vi "SEC code V4.9.vi"() -> ()   [LabVIEW 2022 SP3]
uses:
  SEC code V3.1/Drivers and Aux files/user.lib/atmcd32d.llb/Shutter_type typedef.ctl
  C:/Users/Benj/Desktop/SEC Software V4.9/EcoChemie.Autolab.Sdk.dll
  EcoChemie.Autolab.Sdk.dll
  SEC code V3.1/Drivers and Aux files/State.ctl
  SEC code V3.1/Drivers and Aux files/SECenumctl.ctl
  SEC code V3.1/Drivers and Aux files/user.lib/atmcd32d.llb/TriggerMode_mode typedef.ctl
  SEC code V3.1/Drivers and Aux files/OSSPEC.ctl
  SEC code V3.1/Drivers and Aux files/OSPEC-enum.ctl
  Labview/IVIUM/IVIUM_remdriver.lvlib
panel:
  out "Current PD 2":dbl
  out "POtential PD 2":dbl
  in  "Tab Control 5":enum32{"AUTOLAB", "IVIUM", "iDUS", "Kymera"}(tab)
  out "current":dbl
  out "Error after autolab connection?":errorcluster
  out "Autolab Connected?":bool
  out "Voltage":dbl format="%#_3e"
  out "PotentialOverload":bool
  out "Bandwidth":i32
  out "CurrentRange":i32
  out "Mode":i32
  out "Measured voltage":dbl
  out "CurrentOverload":bool
  out "Cell on?":bool
  out "current":dbl caption="Current (A)" format="%_4g"
  out "cell on":bool
  out "V (during measurment)":dbl
  out "Potentiostat Status":string
  out "T reached?":bool
  out "Shut down sequence run?":bool
  out "Curent Temp":i32
  in  "Tab Control 4":T1(tab)
  in  "Use autolab?":bool=TRUE
  in  "Embedded Exe File":path=path "C:/Program Files/Metrohm Autolab/Autolab SDK 2.1/Hardware Setup Files/Adk.x"
  in  "Hardware Setup File":path=path "C:/ProgramData/Metrohm Autolab/13.0/HardwareSetup.AUT55157.xml"
  in  "Bandwidth 2":i32(ring)=2 items=["UltraHigh_Speed", "High_Speed", "High_Stability"]
  in  "Start potential (V)":dbl=0.2
  in  "Stop potential (V)":dbl=0.7
  in  "Increment (V)":dbl=0.05
  in  "Default Potential (V)":dbl=0.2
  in  "Wait before \nspectrum (s)":dbl=0.1
  in  "Equilibration \ntime (s)":u32=5
  in  "Reverse Scan\ndirection":bool
  in  "(update and read)":bool
  in  "Tab Control 3":T2(tab)
  in  "Inetegration\n Time (us)":i32=5000
  in  "Continuous \nStrobe Delay (us)":i32
  in  "Number of averages":i32
  in  "Use iDus?":bool
  in  "Return detector \nto room T?":bool
  in  "Init, Cool, read dark,\nOR\nWarm/de-init detector":bool
  in  "Temperature\n(degrees C)":i32=-80
  in  "Number of scans in kinetic cycle":i32=30
  in  "Exposure time (s)":dbl=0.03
  in  "Tab Control 2":T3(tab)
  in  "V 1 time (s)":dbl=10.0
  in  "V off time":dbl=30.0
  in  "Sampling\n delay (s)":dbl
  in  "V 2 time (s)":dbl=20.0
  in  "Run OSPSEC":bool
  in  "Square wave?":bool
  out "OCP I (close to 0)":dbl
  out "OCP":dbl format="%_3f"
  in  "V1 (V)":dbl=0.4
  in  "V2 (V)":dbl=0.8
  in  "Slow sample time (s)":dbl=1500.0
  out "Time during PD":u32
  in  "File Name":string="test-1"
  in  "File Path":path=path "C:/Users/Benj/Documents/test"
  in  "Tab Control":T4(tab)
  out "?":T5(graph)
  out "?":cluster{i32[], dbl[]}(graph)
  out "?":T5(graph)
  out "?":T5(graph)
  out "Current during PD":dbl(graph)=1.602783203125e-06
  out "?":cluster{dbl[], dbl[]}(graph)
  out "Potential  During PD":dbl(graph)=-0.0002471923828124972
  out "Setpoint":dbl
  out "?":cluster{i32[], "array":i32[]}(graph)
  out "I_overload":bool
  out "Aninput1_overload":bool
  out "E_overload":bool
  out "cell-off button pressed":bool
  in  "Default\nCurrent range":T6(ring)=enum."100 uA"
  in  "Default Filter":T7(ring)=enum."10 kHz"
  out "Device serial number":string
  in  "Set Stability":T8(ring)=enum."Standard"
  out "Number of Spectrometers":i32
  out "IDus not in read loop? (kinetic)":bool
  out "Get status return code":dbl
  out "xpixels":i32
  out "ypixels":i32
  out "Calculated exposure time":sgl format="%.2f"
  out "Check timings return code":u32
  out "Set temprature\nreturn code":u32
  out "get aquired data return code":u32
  out "Start Aquisition return code":u32
  out "Init. return code":u32
  out "Cooler Off return code":u32
  out "Time before the start of current aquisition (ms)":u32
  out "Time  after the aquisition (before fetch data), (ms)":u32
  in  "Shutter opens on TTL":T9=enum."TTL High"
  in  "Shutter open and close time":i32
  out "Get aqisition ok? (kinetic mode)":bool
  out "Time taken to apply V2":u32
  out "Values to re-intialise to at end\nof the measument":T10
  out "V2 applied?":bool
  out "ContinuousStrobe Out":u32
  out "Wrapper Out":u32
  out "WL Values":dbl[](array[numeric])
  out "Number of time the OCEAN averaging loop has run -1":i32
  out "Adc":refnum<k24>
  out "Sampler 2":refnum<k24>
  out "Dio":refnum<k24>
  out "Dac":refnum<k24>
  out "instrument":refnum<k24>
  out "Ei":refnum<k24>
  out "AutolabConnection":refnum<k24>
  out "EI status supported for":string[](array[string])
  out "TemperatureOverload":bool
  out "ManualCellSwitch":bool
  out "Oscillation":bool
  out "PD ENDED\nEXIT MEASURMENT":bool=TRUE
  out "Current PD":dbl
  out "POtential PD":dbl
  in  "Exit and disconnect":bool
  # "Program control"
  # "Potential decay control"
  # "Spectrometer control"
  # "System status"
  # "SEC control"
  # "Cell on?"
  # "Use the integration time program in the same folder as this program\nto get the optimum value. For kinetic mode the time resolution is limited \nby integration time"
  # "Unless you know what you are doing keep these at 0.03 and 30"
  # "I overload overload"
  # "off button pressed"
  # "Aninput1 overload"
  # "E overload"
  # "OSPEC loop exit"
  # "Checklist for avoiding errors:\n(1) Light on the IVIUM should be blue with red flashes\nIf the system crahes and the light is red then connect and disconnect in IVUM soft/turn stat off/on\n(2) Maya Pro should read in ocean view/or the get intensity program\nIf maya is not reading connect and disconnect USB.\n(3) If errors persist rrepeat steps 1 + 2 then re-compile code by clicking the\nwhite (run) whilst holding down CRTL + (left) SHIFT\n(4) IF USING THE iDus DO NOT EXIT WITHOUT WARMING CAMERA BACK TO ROOM T,YOU \nWILL DAMAGE IT \n(6) if the IVIUM.dll does not load click broken arrows and \"show error\" until you see the call library function (see blue circles). Double click on this and paste the following into the directory (red circle):   \n%windir%\\Labview\\IVIUM\\IVIUM_remdriver.dll"
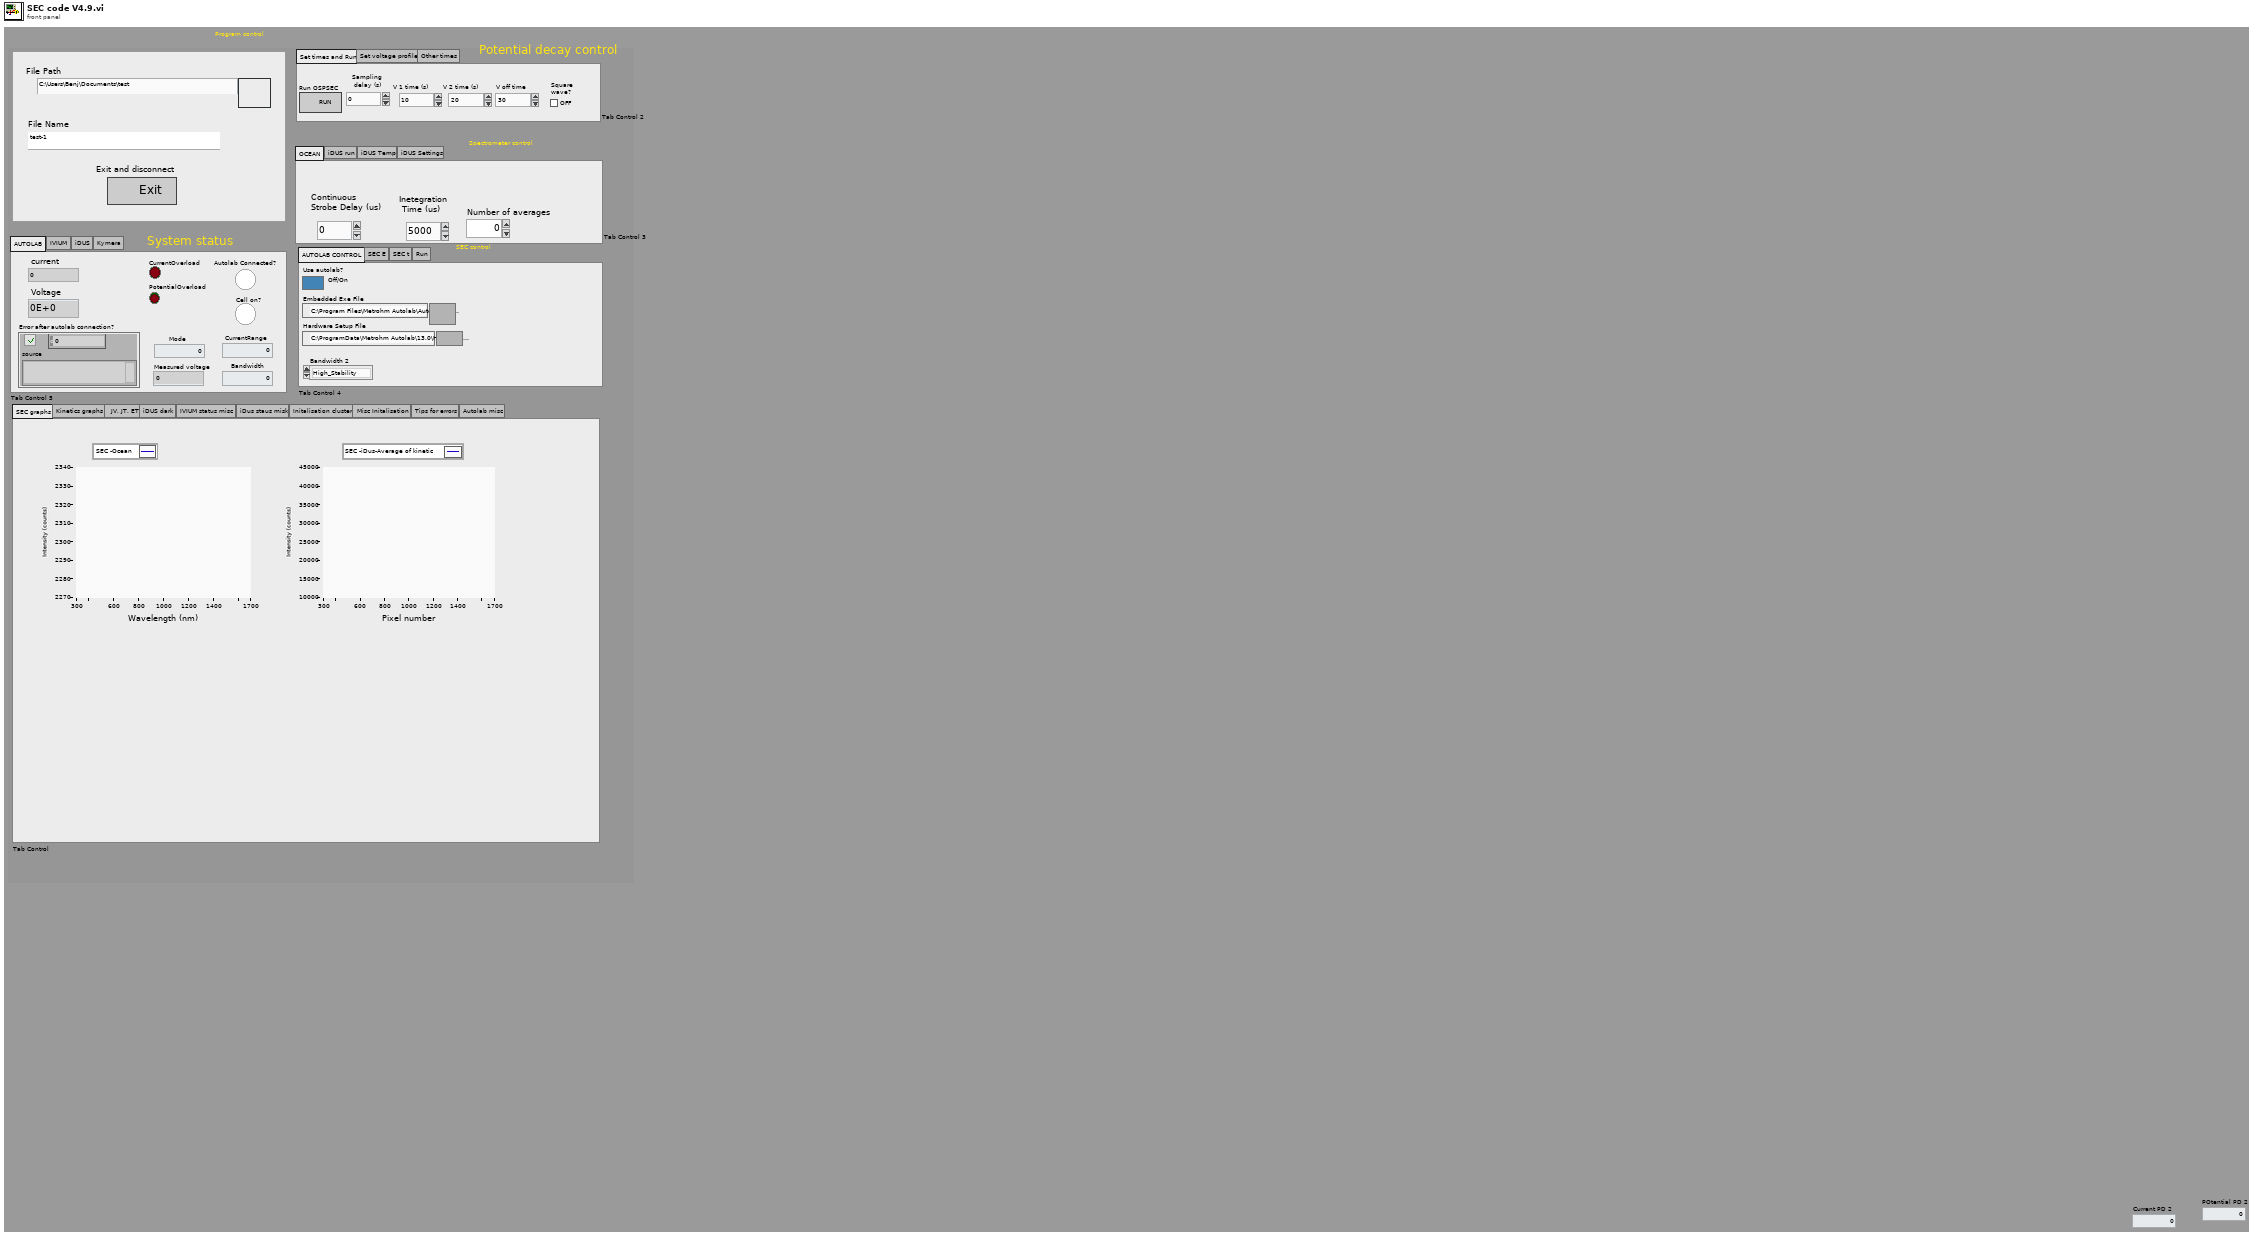
[diagram p1: front panel]
types:
  T1 = enum32{"AUTOLAB CONTROL", "SEC E", "SEC t", "Run"}
  T2 = enum32{"OCEAN", "iDUS run", "iDUS Temp", "iDUS Settings"}
  T3 = enum32{"Set times and Run", "Set voltage profile", "Other times"}
  T4 = enum32{"SEC graphs", "Kinetics graphs", " JV, JT, ET", "iDUS dark", "IVIUM status misc", "iDus staus misk", "Initalisation cluster", "Misc Initalisation ", "Tips for errors", "Autolab misc"}
  T5 = cluster{"WL Values":dbl[], "Spectrum Values":dbl[]}
  T6 = enum16{"10 A", "1 A", "100 mA", "10 mA", "1 mA", "100 uA", "10 uA", "1 uA", "100 nA", "10 nA", "1 nA", "100 pA", "10 pA", "1 pA"}
  T7 = enum16{"1 MHz", "100 kHz", "10 kHz", "1 kHz", "10 Hz"}
  T8 = enum16{"High Speed", "Standard", "High Stability"}
  T9 = typedef "Shutter_type typedef.ctl" = enum16{"TTL Low", "TTL High"}
  T10 = cluster{"Currents":dbl[], "Potentials":dbl[], "Device Status":string, "Device serial no":string, "Current":dbl, "Default \nPotential":dbl, "I overload":bool, "Cell On":bool, "E overload":bool, "Aninput1 overload":bool, "Cell off button pressed":bool, "Start potential":dbl, "Stop potential":dbl, "Increment":dbl, "SEC":dbl[], "Path":path, "File name":string}
  T11 = cluster{"Current array":dbl[], "Potential array":dbl[], "Status":string, "Serial No":string, "Current":dbl, "Default\n potential":dbl, "I overload":bool, "Cell on":bool, "E overload":bool, "Cell of button pressed":bool, "Aninput1 overload":bool, "Stop \npotential":dbl, "Start \npotential":dbl, "Increment":dbl, "Spectrum":dbl[][], "Path":path, "File Name":string, "Sample rate":dbl, "V2 time":dbl, "V off time":dbl, "V 2":dbl, "V 1":dbl, "V1 time":dbl, "Time array":dbl[], "Integration time":i32, "Continous strobe delay":i32, "Time elapsed ":i32, "Start time":i32, "Time for E measurment":i32[], "Time for I measurment ":i32[], "Time for spectrum measurment":i32[], "Return detector to \nroom T":bool, "Number of scans in kinetic cycle":i32, "Exposure time":i32}
  T12 = typedef "State.ctl" = enum16{"Initialize", "Wait for Event", "Run SEC", "Run OSPEC", "Initialse and cool iDus", "Exit"}
  T13 = typedef "SECenumctl.ctl" = enum16{"Read spectrum from Ocean", "Read spectrum from iDus", "Apply potential", "Wait", "Apply potential Autolab"}
  T14 = typedef "TriggerMode_mode typedef.ctl" = enum16{"Internal", "External", "N/A (2)", "N/A (3)", "N/A (4)", "N/A (5)", "External Start", "External Exposure (Bulb)", "N/A (8)", "External FVB EM", "Software", "N/A (11)", "External Charge Shifting"}
  T15 = typedef "OSSPEC.ctl" = enum16{"Read Potential and spectrum", "Read current and spectrum", "Reinitialise Cell", "Apply V1", "End measurment", "Apply V2"}
  T16 = typedef "OSPEC-enum.ctl" = enum16{"Check exit", "Read", "Wait"}
  T17 = enum16{"off", "EStat4EL", "EStat2EL", "EStatDummy1", "EStatDummy2", "EStatDummy3", "EStatDummy4", "IStat4EL", "IStat2EL", "IStatDummy", "BiStat4EL", "BiStat2EL"}
  T18 = typedef "Error Code Enum typedef.ctl" = enum32{"N/A (0)", "DRV_ERROR_CODES", "DRV_SUCCESS", "DRV_VXDNOTINSTALLED", "DRV_ERROR_SCAN", "DRV_ERROR_CHECK_SUM", "DRV_ERROR_FILELOAD", "DRV_UNKNOWN_FUNC", "DRV_ERROR_VXD_INIT", "DRV_ERROR_ADDRESS", "DRV_ERROR_PAGELOCK", "DRV_ERROR_PAGEUNLOCK", "DRV_ERROR_BOARDTEST", "DRV_ERROR_ACK", "DRV_ERROR_UP_FIFO", "DRV_ERROR_PATTERN", "N/A (16)", "DRV_ACQUISITION_ERRORS", "DRV_ACQ_BUFFER", "DRV_ACQ_DOWNFIFO_FULL", "DRV_PROC_UNKONWN_INSTRUCTION", "DRV_ILLEGAL_OP_CODE", "DRV_KINETIC_TIME_NOT_MET", "DRV_ACCUM_TIME_NOT_MET", "DRV_NO_NEW_DATA", "N/A (25)", "DRV_SPOOLERROR", "N/A (27)", "N/A (28)", "N/A (29)", "N/A (30)", "N/A (31)", "N/A (32)", "DRV_TEMPERATURE_CODES", "DRV_TEMPERATURE_OFF", "DRV_TEMPERATURE_NOT_STABILIZED", "DRV_TEMPERATURE_STABILIZED", "DRV_TEMPERATURE_NOT_REACHED", "DRV_TEMPERATURE_OUT_RANGE", "DRV_TEMPERATURE_NOT_SUPPORTED", "DRV_TEMPERATURE_DRIFT", "N/A (41)", "N/A (42)", "N/A (43)", "N/A (44)", "N/A (45)", "N/A (46)", "N/A (47)", "N/A (48)", "DRV_GENERAL_ERRORS", "DRV_INVALID_AUX", "DRV_COF_NOTLOADED", "DRV_FPGAPROG", "DRV_FLEXERROR", "DRV_GPIBERROR", "N/A (55)", "N/A (56)", "N/A (57)", "N/A (58)", "N/A (59)", "N/A (60)", "N/A (61)", "N/A (62)", "N/A (63)", "DRV_DATATYPE", "DRV_DRIVER_ERRORS", "DRV_P1INVALID", "DRV_P2INVALID", "DRV_P3INVALID", "DRV_P4INVALID", "DRV_INIERROR", "DRV_COFERROR", "DRV_ACQUIRING", "DRV_IDLE", "DRV_TEMPCYCLE", "DRV_NOT_INITIALIZED", "DRV_P5INVALID", "DRV_P6INVALID", "DRV_INVALID_MODE", "DRV_INVALID_FILTER", "DRV_I2CERRORS", "DRV_I2CDEVNOTFOUND", "DRV_I2CTIMEOUT", "DRV_P7INVALID", "N/A (84)", "N/A (85)", "N/A (86)", "N/A (87)", "N/A (88)", "N/A (89)", "DRV_IOCERROR", "DRV_VRMVERSIONERROR"}
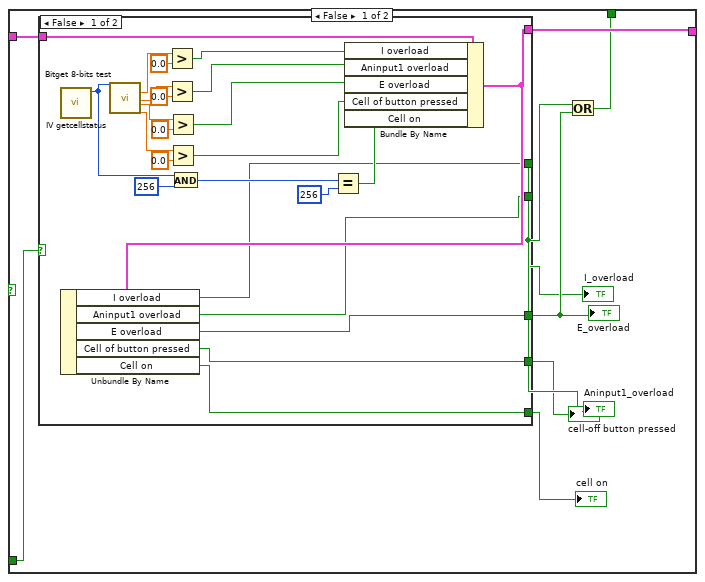
[diagram p2: hidden frame]
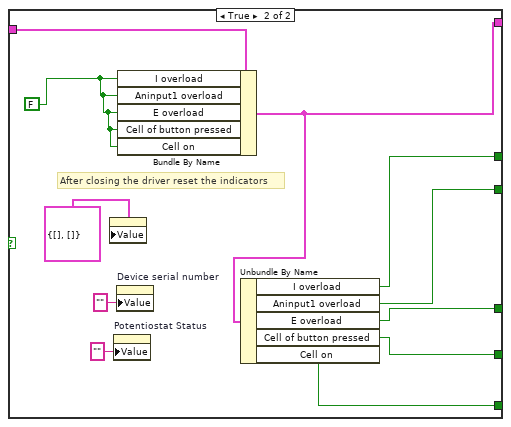
[diagram p3: hidden frame]
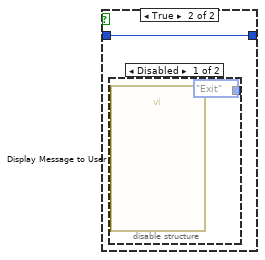
[diagram p4: hidden frame]
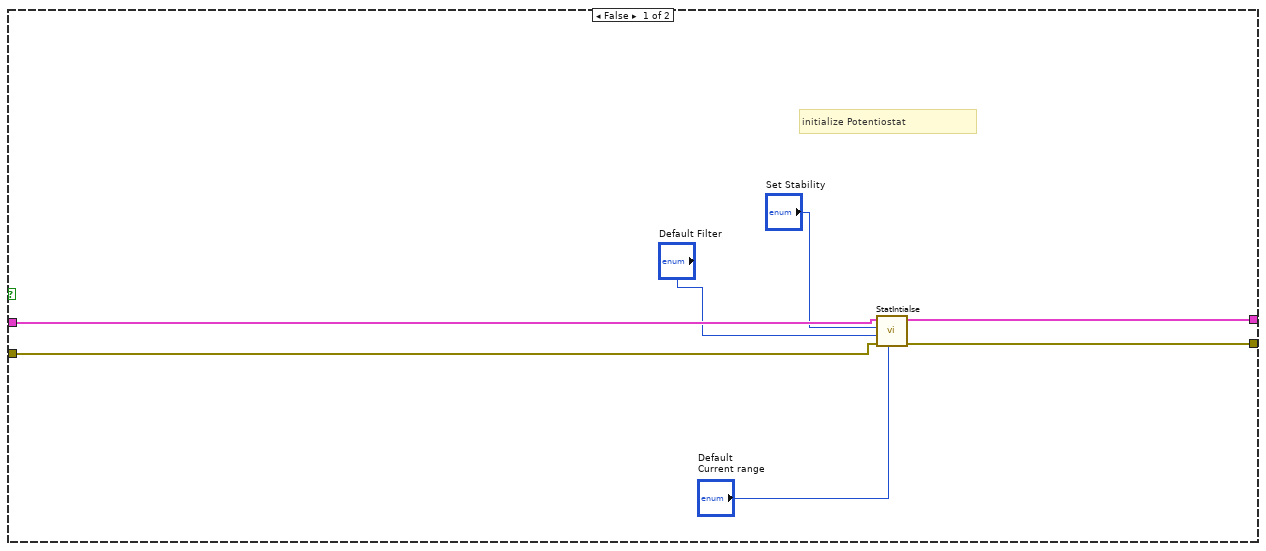
[diagram p7: hidden frame]
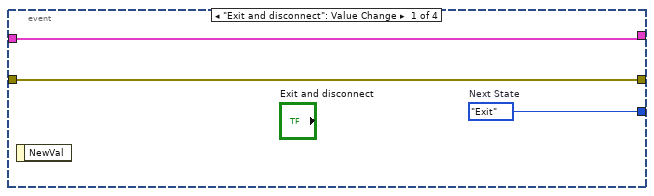
[diagram p9: hidden frame]
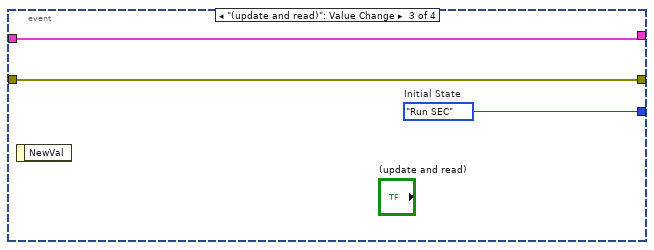
[diagram p10: hidden frame]
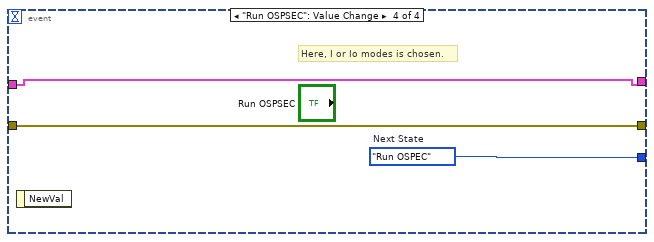
[diagram p11: hidden frame]
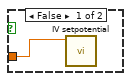
[diagram p12: hidden frame]
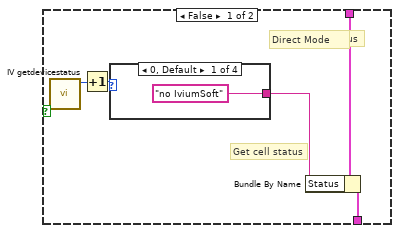
[diagram p13: hidden frame]
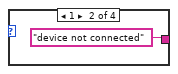
[diagram p14: hidden frame]
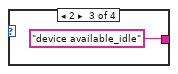
[diagram p15: hidden frame]
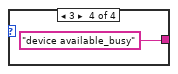
[diagram p16: hidden frame]
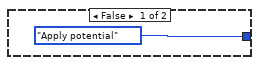
[diagram p17: hidden frame]
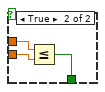
[diagram p20: hidden frame]
diagram:
  w1 = T11 {"Current array"=[], "Potential array"=[], "Status"="", "Serial No"="", "Current"=0.0, "Default\n potential"=0.0, "I overload"=FALSE, "Cell on"=FALSE, "E overload"=FALSE, "Cell of button pressed"=FALSE, "Aninput1 overload"=FALSE, "Stop \npotential"=0.0, "Start \npotential"=0.0, "Increment"=0.0, "Spectrum"=[], "Path"=path "", "File Name"="", "Sample rate"=0.0, "V2 time"=0.0, "V off time"=0.0, "V 2"=0.0, "V 1"=0.0, "V1 time"=0.0, "Time array"=[], "Integration time"=0, "Continous strobe delay"=0, "Time elapsed "=0, "Start time"=0, "Time for E measurment"=[], "Time for I measurment "=[], "Time for spectrum measurment"=[], "Return detector to \nroom T"=FALSE, "Number of scans in kinetic cycle"=0, "Exposure time"=0}  # Init cluster
  w3 = State."Initialize"  # Initial State
  n1 = while {
    shift-right: [w21] -> _
    shift-left: w3 -> [w38]
    shift-right: [w24] -> _
    shift-left: w1 -> [w17]
    shift-right: [w25] -> _
    shift-left: errorcluster {"status"=FALSE, "code"=0, "source"=""} ("error constant") -> [w37]
    stop <- w35 stop-if-true
    # "Main VI State Machine"
    n2 = Bundle By Name(cluster=w17, "Sample rate"="Sampling\n delay (s)", "V1 time"="V 1 time (s)", "V2 time"="V 2 time (s)", "V off time"="V off time", "V 2"="V2 (V)", "V 1"="V1 (V)", "Integration time"="Inetegration\n Time (us)", "Continous strobe delay"="Continuous \nStrobe Delay (us)", "Exposure time"="Exposure time (s)", "Number of scans in kinetic cycle"="Number of scans in kinetic cycle") -> (w11:T11)
    n3 = Bundle By Name(cluster=w11, "Default\n potential"="Default Potential (V)", "Start \npotential"="Start potential (V)", "Stop \npotential"="Stop potential (V)", "Increment"="Increment (V)", "Path"="File Path", "File Name"="File Name") -> (w23:T11)
    n4 = case shown="\"Run SEC\"" w38 {
      tunnel: [w94 w137 w185 w504 w544 w1701] -> w7
      tunnel: [w93 w134 FALSE ("Stop Loop?") w501 FALSE ("Stop Loop?") _] -> w36
      tunnel: w23 -> [w91 w131 w174 w505 w543 w1699]
      tunnel: [w90 w132 w159 w505 w539 w1699] -> w31
      tunnel: w37 -> [w95 w136 w183 w507 w541 w1698]
      tunnel: [w96 w135 w182 w508 w540 w1698] -> w25
      tunnel: [1 ("devconnect") 1 ("devconnect") 1 ("devconnect") w506 1 ("devconnect") 1 ("devconnect")] -> w22
      frame "Initialize" {
        w93 = FALSE  # Stop Loop?
        w94 = State."Wait for Event"  # Next State
        # "Initialize - Initialize variables needed"
        n5 = case shown="True" "Use autolab?" {
          tunnel: [w104 w108] -> w96
          tunnel: w95 -> [w103 _]
          tunnel: w91 -> [w102 w130]
          tunnel: [w98 w130] -> w90
          frame False {
            # "initialize Potentiostat"
            n6 = call "StatIntialse.vi"("Init cluster 2"=w102, "Set Stability"="Set Stability", "Default\n Filter"="Default Filter", "error in (no error)"=w103, "Default\nCurrent range"="Default\nCurrent range") -> ("Init cluster"=w98:T11, "error out"=w104:errorcluster)  [unwired: 4 in]
          }
          frame True {
            w111 = 0 items=["Potentiostatic", "Galvanostatic"] ("Mode")
            w112 = -3 items=["CR07_1A"=0, "CR06_10A"=1, "CR01_100A"=2, "CR00_1000A"=3, "CR05_20A"=20, "CR04_40A"=40, "CR03_50A"=60, "CR02_80A"=80, "CR19_1pA"=-12, "CR18_10pA"=-11, "CR17_100pA"=-10, "CR16_1nA"=-9, "CR15_10nA"=-8, "CR14_100nA"=-7, "CR13_1uA"=-6, "CR12_10uA"=-5, "CR11_100uA"=-4, "CR10_1mA"=-3, "CR09_10mA"=-2, "CR08_100mA"=-1] ("CurrentRange")
            w114 = 1 items=["Off", "On"] ("CellOnOff")
            n7 = call "Connect AutoLab.vi"("Embedded Exe File"="Embedded Exe File", "Hardware Setup File"="Hardware Setup File") -> ("error out"=w119:errorcluster, ".NET Refnum out"=w128:refnum<k24>)  [unwired: 8 in]
            "Error after autolab connection?" <- w119
            n8 = property class="Instrument"(reference=w128, error in=w119) -> (reference out=→"instrument":refnum<k24>, error out=w120:errorcluster, "Adc"=→"Adc":refnum<k24>, "Dac"=→"Dac":refnum<k24>, "Dio"=→"Dio":refnum<k24>, "AutolabConnection"=w116:refnum<k24>, "Ei"=w107:refnum<k24>)
            "AutolabConnection" <- w116
            n9 = property class="AutolabConnection"(reference=w116) -> ("IsConnected"=→"Autolab Connected?":bool)  [unwired: 1 in, 2 out]
            n10 = property class="EI"(reference=w107, error in=w120) -> (reference out=→"Ei":refnum<k24>, error out=w127:errorcluster, "Sampler"=→"Sampler 2":refnum<k24>)
            n11 = property on="Bandwidth 2" class="Ring (strict)"() -> ("Value"=w113:i32)  [unwired: 2 in, 2 out]
            n12 = property on="Default Potential (V)" class="DigNum (strict)"() -> ("Value"=w110:dbl)  [unwired: 2 in, 2 out]
            n13 = Build Array(w120, w127) -> (w121:errorcluster[])
            n14 = Merge Errors(w121) -> (w109:errorcluster)
            n15 = property class="EI"(reference=w107, error in=w109, "Bandwidth"=w113, "CellOnOff"=w114, "CurrentRange"=w112, "Mode"=w111, "Setpoint"=w110) -> (error out=w108:errorcluster, "Current"=w106:dbl, "Potential"=w105:dbl)  [unwired: 1 out]
            n16 = property on="current" class="DigNum (strict)"("Value"=w106) -> ()  [unwired: 2 in, 2 out]
            n17 = property on="Voltage" class="DigNum (strict)"("Value"=w105) -> ()  [unwired: 2 in, 2 out]
          }
        }
        n18 = property on="V2 applied?" class="Bool (strict)"("Value"=FALSE ("V2 applied")) -> ()  [unwired: 2 in, 2 out]
        "Values to re-intialise to at end\nof the measument" <- T10 {"Currents"=[], "Potentials"=[], "Device Status"="", "Device serial no"="", "Current"=0.0, "Default \nPotential"=0.0, "I overload"=FALSE, "Cell On"=FALSE, "E overload"=FALSE, "Aninput1 overload"=FALSE, "Cell off button pressed"=FALSE, "Start potential"=0.0, "Stop potential"=0.0, "Increment"=0.0, "SEC"=[], "Path"=path "", "File name"=""} ("Values to re-intialise to at end\nof the measument")
      }
      frame "Wait for Event" {
        w134 = FALSE  # Stop Loop?
        # "Wait for Event - Use an Event Structure to monitor the user interface for events that run different states of the state machine."
        n19 = event shown="[1] \"Init, Cool, read dark, OR Warm/de-init detector\": Value Change" {
          selector: _ -> [_ _ _ _]
          dyn-events: _ -> [_ _ _ _]
          timeout: _ -> [_ _ _ _]
          tunnel: [w140 State."Initialse and cool iDus" ("Next State") w147 w151] -> w137
          tunnel: w136 -> [w139 w145 w148 w150]
          tunnel: [w139 w145 w148 w150] -> w135
          tunnel: w131 -> [w138 w143 w146 w149]
          tunnel: [w138 w141 w146 w149] -> w132
          event "Exit and disconnect": Value Change {
            w140 = State."Exit"  # Next State
            n20 = event-data() -> ()  [unwired: 1 in, 1 out]
          }
          event "Init, Cool, read dark,\nOR\nWarm/de-init detector": Value Change {
            n21 = event-data() -> ()  [unwired: 1 in, 4 out]
            n22 = Bundle By Name(cluster=w143, "Return detector to \nroom T"="Return detector \nto room T?") -> (w141:T11)
          }
          event "(update and read)": Value Change {
            w147 = State."Run SEC"  # Initial State
            n23 = event-data() -> ()  [unwired: 1 in, 1 out]
          }
          event "Run OSPSEC": Value Change {
            w151 = State."Run OSPEC"  # Next State
            # "Here, I or Io modes is chosen."
            n24 = event-data() -> ()  [unwired: 1 in, 1 out]
          }
        }
      }
      frame "Run SEC" {
        w185 = State."Wait for Event"  # Next State
        n25 = property on="Use autolab?" class="Bool (strict)"() -> ("Value"=w154:bool)  [unwired: 2 in, 2 out]
        n26 = case shown="True" w154 {
          tunnel: w174 -> [w191 w199]
          tunnel: [w190 w199] -> w161
          frame False {
            # "Get cell status"
            # "Get Device Status"
            # "Direct Mode"
            n27 = call "IV getdevicestatus.vi"() -> ("return type"=w193:i32)  [unwired: 10 in, 1 out]
            n28 = Increment(x=w193) -> (x+1=w192:i32)
            n29 = case shown="0, Default" w192 {
              tunnel: ["no IviumSoft" "device not connected" "device available_idle" "device available_busy"] -> w194
              frame 0, Default {
              }
              frame 1 {
              }
              frame 2 {
              }
              frame 3 {
              }
            }
            n30 = Bundle By Name(cluster=w191, "Status"=w194) -> (w190:T11)
          }
          frame True {
          }
        }
        n31 = property on="Use autolab?" class="Bool (strict)"() -> ("Value"=w156:bool)  [unwired: 2 in, 2 out]
        n32 = case shown="True" w156 {
          tunnel: [SECenumctl."Apply potential" SECenumctl."Apply potential Autolab"] -> w181
          frame False {
          }
          frame True {
          }
        }
        n33 = Unbundle By Name(w161) -> ("Increment"=w180:dbl, "Start \npotential"=w184:dbl, "Stop \npotential"=w175:dbl)
        n34 = while {
          shift-right: [w227] -> w158
          shift-left: w161 -> [w228]
          tunnel: w180 -> [w223]
          tunnel: w184 -> [w222]
          shift-right: [w224] -> w182
          shift-left: w183 -> [w225]
          shift-right: [w216] -> _
          shift-left: w181 -> [w220]
          shift-right: [w218] -> w160
          shift-left: dbl[] [0.0] -> [w217]
          shift-right: [w213] -> w164
          shift-left: dbl[] [0.0] -> [w214]
          tunnel: w175 -> [w215]
          shift-right: [w212] -> w173
          shift-left: dbl[][] [] -> [w211]
          tunnel: "Reverse Scan\ndirection" -> [w210]
          tunnel: [w208] -> _
          tunnel: [w208] -> _
          shift-right: [w207] -> _
          shift-left: -3 ("y") -> [w206]
          i -> [w226]
          stop <- w208 stop-if-true
          n35 = case shown="\"Read spectrum from Ocean\"" w220 {
            tunnel: w228 -> [w251 w315 w350 w365 w463]
            tunnel: [w250 w314 w350 w365 w463] -> w227
            tunnel: w226 -> [w264 w324 _ w372 w471]
            tunnel: w225 -> [w261 w306 w346 w374 w472]
            tunnel: [w252 w295 w346 w374 w472] -> w224
            tunnel: w223 -> [w247 w312 _ _ _]
            tunnel: w222 -> [w263 w323 _ _ _]
            tunnel: [w244 w307 w349 w378 w477] -> w221
            tunnel: [w236 w310 w348 w377 w476] -> w219
            tunnel: [w255 w318 w347 w379 w475] -> w218
            tunnel: w217 -> [w256 w319 w347 w379 w475]
            tunnel: [SECenumctl."Wait" SECenumctl."Wait" w351 w360 w459] -> w216
            tunnel: w215 -> [w236 w310 _ _ _]
            tunnel: w214 -> [w254 w317 w342 w380 w473]
            tunnel: [w253 w316 w342 w380 w473] -> w213
            tunnel: [w248 w313 w341 w368 w466] -> w212
            tunnel: w211 -> [w248 w313 w341 w369 w465]
            tunnel: w210 -> [w237 w311 w340 w376 w464]
            tunnel: [w237 w311 w339 w375 w464] -> w209
            tunnel: w206 -> [w235 w305 w337 w362 w460]
            tunnel: [w235 w304 w337 w362 w460] -> w207
            frame "Apply potential", Default {
              # "Here, the while loop iterates three times for every one change of potential. The loop counter is therefore diveded by three, multipled by the increment and then added to the start  potential to give the next potential in the LSV. Potential is applied, then current is read. These go into a build array function . A wait is inclided to alow the sample to equilibriate at the start potential"
              n36 = Divide(x=w264, y=3) -> (x/y=w259:dbl)
              n37 = Multiply(x=w247, y=w259) -> (x*y=w262:dbl)
              n38 = Add(x=w262, y=w263) -> (x+y=w244:dbl)
              "V (during measurment)" <- w244
              n39 = call "IV setpotential.vi"("error in (no error)"=w261, "value"=w244) -> ("error out"=w258:errorcluster)  [unwired: 7 in, 2 out]
              n40 = Equal To 0?(x=w259) -> (x = 0?=w260:bool)
              n41 = case shown="True" w260 {
                tunnel: w258 -> [w274 w276]
                tunnel: [w274 w276] -> w257
                frame False {
                }
                frame True {
                  n42 = Multiply(x=u32 1000, y="Equilibration \ntime (s)") -> (x*y=w275:u32)
                  n43 = Wait (ms)(milliseconds to wait=w275) -> ()  [unwired: 1 out]
                }
              }
              n44 = Equal To 0?(x=w247) -> (x = 0?=w242:bool)
              n45 = Absolute Value(x=w244) -> (abs(x)=w245:dbl)
              n46 = Build Array (concatenate)(w244, w256) -> (w255:dbl[])
              n47 = Greater?(x=w245, y=3.0) -> (0:w243:bool)
              n48 = call "IV getcurrent.vi"("error in (no error)"=w257) -> ("error out"=w240:errorcluster, "value out"=w238:dbl)  [unwired: 8 in, 1 out]
              n49 = Or(x=w242, y=w243) -> (x .or. y?=w241:bool)
              n50 = flat-sequence {
                tunnel: w240 -> [w268]
                tunnel: [w268] -> w239
                tunnel: w238 -> [w267]
                frame #0 {
                  n51 = call "Current ranging routine (SubVI).vi"("Current"=w267) -> ()  [unwired: 11 in]
                  n52 = Wait (ms)(milliseconds to wait=u32 100) -> ()  [unwired: 1 out]
                }
              }
              n53 = case shown="True" w241 {
                frame False {
                }
                frame True {
                  # "abort if E >3 V or\ndelta E =0"
                  n54 = call "IV setcellon.vi"("cellon"=0) -> ("error out"=w272:errorcluster)  [unwired: 8 in, 2 out]
                  n55 = call "IV close.vi"("error in (no error)"=w272) -> ("error out"=w270:errorcluster)  [unwired: 9 in, 1 out]
                  n56 = call "Display Message to User2"("error in (no error)"=w270) -> ("OK"=w273:bool)  [unwired: 9 in, 1 out]
                  n57 = Stop(stop? (T)=w273) -> ()
                }
              }
              n58 = call "IV getcurrent.vi"("error in (no error)"=w239) -> ("error out"=w252:errorcluster, "value out"=w249:dbl)  [unwired: 8 in, 1 out]
              n59 = Bundle By Name(cluster=w251, "Current"=w249) -> (w250:T11)
              n60 = property on="current" class="DigNum (strict)"("Value"=w249) -> ()  [unwired: 2 in, 2 out]
              n61 = Build Array (concatenate)(w249, w254) -> (w253:dbl[])
            }
            frame "Apply potential Autolab" {
              w308 = 1 items=["Off", "On"] ("CellOnOff")
              w303 = 0 items=["Potentiostatic", "Galvanostatic"] ("Mode")
              # "Here, the while loop iterates three times for every one change of potential. The loop counter is therefore diveded by three, multipled by the increment and then added to the start  potential to give the next potential in the LSV. Potential is applied, then current is read. These go into a build array function . A wait is inclided to alow the sample to equilibriate at the start potential"
              n62 = Divide(x=w324, y=3) -> (x/y=w320:dbl)
              n63 = Multiply(x=w312, y=w320) -> (x*y=w322:dbl)
              n64 = Add(x=w322, y=w323) -> (x+y=w307:dbl)
              "Voltage" <- w307
              n65 = property on="Ei" class="Ref (strict)"() -> ("Value"=w282:refnum<k24>)  [unwired: 2 in, 2 out]
              n66 = property class="EI"(reference=w282, error in=w306, "Bandwidth"="Bandwidth 2", "CellOnOff"=w308, "CurrentRange"=w305, "Mode"=w303, "Setpoint"=w307) -> (error out=w287:errorcluster)  [unwired: 1 out]
              n67 = Equal To 0?(x=w320) -> (x = 0?=w321:bool)
              n68 = case shown="False" w321 {
                tunnel: w287 -> [w332 w335]
                tunnel: [w332 w335] -> w299
                frame False {
                }
                frame True {
                  n69 = property on="Equilibration \ntime (s)" class="DigNum (strict)"() -> ("Value"=w333:u32)  [unwired: 2 in, 2 out]
                  n70 = Multiply(x=u32 1000, y=w333) -> (x*y=w334:u32)
                  n71 = Wait (ms)(milliseconds to wait=w334) -> ()  [unwired: 1 out]
                }
              }
              n72 = property on="Sampler 2" class="Ref (strict)"() -> ("Value"=w280:refnum<k24>)  [unwired: 2 in, 2 out]
              n73 = property class="EI"(reference=w282, error in=w287) -> (error out=w286:errorcluster, "EiStatusSupportedFor"=→"EI status supported for":string[])  [unwired: 1 out]
              n74 = invoke class="Sampler" method="Sample"(reference=w280, error in=w287) -> (error out=w285:errorcluster)  [unwired: 1 in, 2 out]
              n75 = Build Array (concatenate)(w307, w319) -> (w318:dbl[])
              n76 = property class="EI"(reference=w282, error in=w299) -> (reference out=w281:refnum<k24>, error out=w298:errorcluster, "Bandwidth"=→"Bandwidth":i32, "CurrentRange"=→"CurrentRange":i32, "Mode"=→"Mode":i32, "Setpoint"=w296:dbl, "Current"=w297:dbl)
              "Measured voltage" <- w296
              n77 = flat-sequence {
                tunnel: w298 -> [w330]
                tunnel: [w330] -> w284
                tunnel: [w329] -> w304
                tunnel: w297 -> [w328]
                tunnel: w296 -> [w327]
                frame #0 {
                  n78 = Wait (ms)(milliseconds to wait=u32 100) -> ()  [unwired: 1 out]
                  n79 = call "Range_selector.vi"("potential"=w327, "current"=w328) -> ("range integer"=w329:i32)  [unwired: 9 in]
                }
              }
              n80 = Merge Errors(w284, w286, w285) -> (w283:errorcluster)
              n81 = call "P_Stat_Status1.vi"("error in (no error)"=w283, ".NET Refnum in"=w281) -> ("error out"=w289:errorcluster, "ManualCellSwitch"=→"ManualCellSwitch":bool, "Oscillation"=→"Oscillation":bool, "TemperatureOverload"=→"TemperatureOverload":bool, "CurrentOverload"=→"CurrentOverload":bool, "Cell"=→"Cell on?":bool)  [unwired: 3 in, 1 out]
              n82 = property class="EI"(reference=w281, error in=w289) -> (error out=w295:errorcluster, "Current"=w279:dbl)  [unwired: 1 out]
              "current" <- w279
              n83 = Bundle By Name(cluster=w315, "Current"=w279) -> (w314:T11)
              n84 = property on="current" class="DigNum (strict)"("Value"=w279) -> ()  [unwired: 2 in, 2 out]
              n85 = Build Array (concatenate)(w279, w317) -> (w316:dbl[])
            }
            frame "Wait" {
              n86 = Multiply(x="Wait before \nspectrum (s)", y=1000.0) -> (x*y=w345:dbl)
              n87 = Wait (ms)(milliseconds to wait=w345) -> ()  [unwired: 1 out]
              n88 = case shown="False" "Use iDus?" {
                tunnel: [SECenumctl."Read spectrum from Ocean" SECenumctl."Read spectrum from iDus"] -> w351
                frame False {
                }
                frame True {
                }
              }
              n89 = case shown="False" w340 {
                selector: w340 -> [w354 w357]
                tunnel: [0.0 1.0] -> w349
                tunnel: [1.0 ("Stop \npotential") 0.0 ("Stop \npotential")] -> w348
                tunnel: [w354 w357] -> w339
                frame False {
                }
                frame True {
                }
              }
            }
            frame "Read spectrum from iDus" {
              n90 = Unbundle By Name(w365) -> ("Exposure time"=w373:i32, "Number of scans in kinetic cycle"=w366:i32)
              n91 = Equal?(x=w372, y=2) -> (x = y?=w370:bool)
              n92 = Multiply(x=1024, y=w366) -> (x*y=w383:i32)
              n93 = stacked-sequence {
                seq-local: [_ _ _ _ _ _ _ _ _ _ w416 _] -> [_ _ _ _ _ _ _ _ _ _ _ w425]
                tunnel: [_ _ _ _ _ _ _ _ _ _ _ w426] -> w381
                tunnel: w366 -> [_ _ _ _ _ w405 _ _ _ _ _ w424]
                tunnel: w383 -> [_ _ _ _ _ _ _ _ _ _ w417 _]
                tunnel: w373 -> [_ _ _ w401 _ _ _ _ _ _ _ _]
                frame #0 {
                  w398 = u16 3  # AcquisitionMode
                  n94 = call "SetAcquisitionMode.vi"("mode"=w398) -> ()  [unwired: 1 in, 2 out]
                }
                frame #1 {
                  w399 = u16 0  # ReadMode
                  n95 = call "SetReadMode.vi"("mode"=w399) -> ()  [unwired: 1 in, 2 out]
                }
                frame #2 {
                  n96 = call "SetTriggerMode.vi"("mode"=TriggerMode_mode_typedef."Internal") -> ()  [unwired: 1 in, 2 out]
                }
                frame #3 {
                  n97 = call "SetExposureTime.vi"("time"=w401) -> ()  [unwired: 1 in, 2 out]
                }
                frame #4 {
                  n98 = call "GetNumberVSSpeeds.vi"() -> ("number"=w404:i32)  [unwired: 3 in, 2 out]
                  n99 = Subtract(x=w404, y=1) -> (x-y=w402:i32)
                  n100 = call "SetVSSpeed.vi"("index"=w402) -> ()  [unwired: 1 in, 2 out]
                }
                frame #5 {
                  n101 = call "SetNumberKinetics.vi"("number"=w405) -> ()  [unwired: 1 in, 2 out]
                }
                frame #6 {
                  w409 = 0  # Auto Shutter
                  n102 = call "SetShutter.vi"("type"=Shutter_type_typedef."TTL High", "mode"=w409, "closingtime"=0, "openingtime"=0) -> ()  [unwired: 10 in, 2 out]
                }
                frame #7 {
                  n103 = call "GetAcquisitionTimings.vi"() -> ("exposure"=w410:sgl)  [unwired: 11 in, 4 out]
                  n104 = property on="Calculated exposure time" class="DigNum (strict)"("Value"=w410) -> ()  [unwired: 2 in, 2 out]
                }
                frame #8 {
                  n105 = call "StartAcquisition.vi"() -> ("DLL error code"=w411:u32)  [unwired: 2 in, 1 out]
                  n106 = property on="Start Aquisition return code" class="DigNum (strict)"("Value"=w411) -> ()  [unwired: 2 in, 2 out]
                }
                frame #9 {
                  n107 = while {
                    stop <- w414 continue-if-true
                    w415 = u16 72  # DRV ACQUIRING
                    n108 = call "GetStatus.vi"() -> ("DLL error code"=→"Get status return code":u32, "status"=w413:T18)  [unwired: 3 in, 1 out]
                    n109 = Equal?(x=w413, y=w415) -> (x = y?=w414:bool)
                  }
                }
                frame #10 {
                  n110 = flat-sequence {
                    tunnel: [w419] -> w418
                    tunnel: w417 -> [w419]
                    tunnel: [w423] -> w416
                    tunnel: w418 -> [w421]
                    frame #0 {
                    }
                    frame #1 {
                      n111 = call "GetAcquiredData.vi"("size"=w421) -> ("DLL error code"=w420:u32, "array"=w423:i32[])  [unwired: 2 in, 1 out]
                      n112 = Equal?(x=20002 ("DRV_SUCCESS"), y=w420) -> ()  [unwired: 1 out]
                      n113 = property on="get aquired data return code" class="DigNum (strict)"("Value"=w420) -> ()  [unwired: 2 in, 2 out]
                    }
                  }
                }
                frame #11 {
                  n114 = for {
                    N: w424 -> [_]
                    shift-right: [w428] -> w426
                    shift-left: i32[][] [] -> [w430]
                    tunnel: w425 -> [w429]
                    i -> [w433]
                    w431 = 1024 ("x")
                    n115 = Multiply(x=w431, y=w433) -> (x*y=w435:i32)
                    n116 = Equal To 0?(x=w433) -> (x = 0?=w434:bool)
                    n117 = Array Subset(array=w429, index=w435, length=w431) -> (w432:i32[])
                    n118 = case shown="False" w434 {
                      tunnel: w432 -> [w437 w440]
                      tunnel: w430 -> [w438 _]
                      tunnel: [w436 w439] -> w428
                      frame False {
                        n119 = Build Array (concatenate)(w438, w437) -> (w436:i32[][])
                      }
                      frame True {
                        n120 = Build Array(w440) -> (w439:i32[][])
                      }
                    }
                  }
                }
              }
              n121 = property on="Use autolab?" class="Bool (strict)"() -> ("Value"=w361:bool)  [unwired: 2 in, 2 out]
              n122 = case shown="True" w361 {
                tunnel: [SECenumctl."Apply potential" SECenumctl."Apply potential Autolab"] -> w360
                frame False {
                }
                frame True {
                }
              }
              n123 = Unbundle By Name(w365) -> ("Number of scans in kinetic cycle"=w367:i32)
              n124 = flat-sequence {
                tunnel: [w446] -> w363
                tunnel: w381 -> [w444]
                tunnel: w367 -> [w443]
                tunnel: [w441] -> w364
                frame #0 {
                  n125 = for {
                    N: 1023 -> [_]
                    tunnel: w444 -> [w451]
                    tunnel: [w452] -> w446 mode=indexing
                    tunnel: w443 -> [w449]
                    tunnel: [w447] -> w441 mode=indexing
                    i -> [w448]
                    n126 = Index Array(array=w451, index (col)=w448) -> (element=w450:i32[])  [unwired: 1 in]
                    n127 = Add Array Elements(numeric array=w450) -> (sum=w453:i32)
                    n128 = Increment(x=w448) -> (x+1=w447:i32)
                    n129 = Divide(x=w453, y=w449) -> (x/y=w452:dbl)
                  }
                  n130 = Bundle(w441, w446) -> (→"?":cluster{i32[], dbl[]})  [unwired: 1 in]
                }
              }
              n131 = case shown="True" w370 {
                tunnel: w369 -> [w388 _]
                tunnel: w363 -> [w387 w390]
                tunnel: [w386 w391] -> w368
                tunnel: w364 -> [_ w389]
                frame False {
                  n132 = Build Array (concatenate)(w388, w387) -> (w386:dbl[][])
                }
                frame True {
                  n133 = Build Array(w389, w390) -> (w391:dbl[][])
                }
              }
              n134 = case shown="False" w376 {
                selector: w376 -> [w392 w395]
                tunnel: [0.0 1.0] -> w378
                tunnel: [1.0 ("Stop \npotential") 0.0 ("Stop \npotential")] -> w377
                tunnel: [w392 w395] -> w375
                frame False {
                }
                frame True {
                }
              }
            }
            frame "Read spectrum from Ocean" {
              # "Building an matric of WL + intensities of multiple expts"
              n135 = Unbundle By Name(w463) -> ("Integration time"=w462:i32, "Continous strobe delay"=w461:i32)
              n136 = Equal?(x=w471, y=2) -> (x = y?=w469:bool)
              n137 = for {
                N: "Number of averages" -> [_]
                tunnel: [w485] -> w474
                tunnel: [w484] -> w468
                tunnel: w462 -> [w483]
                tunnel: w461 -> [w482]
                shift-right: [w479] -> w457
                shift-left: dbl[] [0.0, 0.0, 0.0, 0.0, 0.0, 0.0, 0.0, 0.0, 0.0, 0.0, 0.0, 0.0, 0.0, 0.0, 0.0, 0.0, 0.0, 0.0, 0.0, 0.0, 0.0, 0.0, 0.0, 0.0, 0.0, 0.0, 0.0, 0.0, 0.0, 0.0, 0.0, 0.0, 0.0, 0.0, 0.0, 0.0, 0.0, 0.0, 0.0, 0.0, 0.0, 0.0, 0.0, 0.0, 0.0, 0.0, 0.0, 0.0, 0.0, 0.0, 0.0, 0.0, 0.0, 0.0, 0.0, 0.0, 0.0, 0.0, 0.0, 0.0, 0.0, 0.0, 0.0, 0.0, 0.0, 0.0, 0.0, 0.0, 0.0, 0.0, 0.0, 0.0, 0.0, 0.0, 0.0, 0.0, 0.0, 0.0, 0.0, 0.0, 0.0, 0.0, 0.0, 0.0, 0.0, 0.0, 0.0, 0.0, 0.0, 0.0, 0.0, 0.0, 0.0, 0.0, 0.0, 0.0, 0.0, 0.0, 0.0, 0.0, 0.0, 0.0, 0.0, 0.0, 0.0, 0.0, 0.0, 0.0, 0.0, 0.0, 0.0, 0.0, 0.0, 0.0, 0.0, 0.0, 0.0, 0.0, 0.0, 0.0, 0.0, 0.0, 0.0, 0.0, 0.0, 0.0, 0.0, 0.0, 0.0, 0.0, 0.0, 0.0, 0.0, 0.0, 0.0, 0.0, 0.0, 0.0, 0.0, 0.0, 0.0, 0.0, 0.0, 0.0, 0.0, 0.0, 0.0, 0.0, 0.0, 0.0, 0.0, 0.0, 0.0, 0.0, 0.0, 0.0, 0.0, 0.0, 0.0, 0.0, 0.0, 0.0, 0.0, 0.0, 0.0, 0.0, 0.0, 0.0, 0.0, 0.0, 0.0, 0.0, 0.0, 0.0, 0.0, 0.0, 0.0, 0.0, 0.0, 0.0, 0.0, 0.0, 0.0, 0.0, 0.0, 0.0, 0.0, 0.0, 0.0, 0.0, 0.0, 0.0, 0.0, 0.0, 0.0, 0.0, 0.0, 0.0, 0.0, 0.0, 0.0, 0.0, 0.0, 0.0, 0.0, 0.0, 0.0, 0.0, 0.0, 0.0, 0.0, 0.0, 0.0, 0.0, 0.0, 0.0, 0.0, 0.0, 0.0, 0.0, 0.0, 0.0, 0.0, 0.0, 0.0, 0.0, 0.0, 0.0, 0.0, 0.0, 0.0, 0.0, 0.0, 0.0, 0.0, 0.0, 0.0, 0.0, 0.0, 0.0, 0.0, 0.0, 0.0, 0.0, 0.0, 0.0, 0.0, 0.0, 0.0, 0.0, 0.0, 0.0, 0.0, 0.0, 0.0, 0.0, 0.0, 0.0, 0.0, 0.0, 0.0, 0.0, 0.0, 0.0, 0.0, 0.0, 0.0, 0.0, 0.0, 0.0, 0.0, 0.0, 0.0, 0.0, 0.0, 0.0, 0.0, 0.0, 0.0, 0.0, 0.0, 0.0, 0.0, 0.0, 0.0, 0.0, 0.0, 0.0, 0.0, 0.0, 0.0, 0.0, 0.0, 0.0, 0.0, 0.0, 0.0, 0.0, 0.0, 0.0, 0.0, 0.0, 0.0, 0.0, 0.0, 0.0, 0.0, 0.0, 0.0, 0.0, 0.0, 0.0, 0.0, 0.0, 0.0, 0.0, 0.0, 0.0, 0.0, 0.0, 0.0, 0.0, 0.0, 0.0, 0.0, 0.0, 0.0, 0.0, 0.0, 0.0, 0.0, 0.0, 0.0, 0.0, 0.0, 0.0, 0.0, 0.0, 0.0, 0.0, 0.0, 0.0, 0.0, 0.0, 0.0, 0.0, 0.0, 0.0, 0.0, 0.0, 0.0, 0.0, 0.0, 0.0, 0.0, 0.0, 0.0, 0.0, 0.0, 0.0, 0.0, 0.0, 0.0, 0.0, 0.0, 0.0, 0.0, 0.0, 0.0, 0.0, 0.0, 0.0, 0.0, 0.0, 0.0, 0.0, 0.0, 0.0, 0.0, 0.0, 0.0, 0.0, 0.0, 0.0, 0.0, 0.0, 0.0, 0.0, 0.0, 0.0, 0.0, 0.0, 0.0, 0.0, 0.0, 0.0, 0.0, 0.0, 0.0, 0.0, 0.0, 0.0, 0.0, 0.0, 0.0, 0.0, 0.0, 0.0, 0.0, 0.0, 0.0, 0.0, 0.0, 0.0, 0.0, 0.0, 0.0, 0.0, 0.0, 0.0, 0.0, 0.0, 0.0, 0.0, 0.0, 0.0, 0.0, 0.0, 0.0, 0.0, 0.0, 0.0, 0.0, 0.0, 0.0, 0.0, 0.0, 0.0, 0.0, 0.0, 0.0, 0.0, 0.0, 0.0, 0.0, 0.0, 0.0, 0.0, 0.0, 0.0, 0.0, 0.0, 0.0, 0.0, 0.0, 0.0, 0.0, 0.0, 0.0, 0.0, 0.0, 0.0, 0.0, 0.0, 0.0, 0.0, 0.0, 0.0, 0.0, 0.0, 0.0, 0.0, 0.0, 0.0, 0.0, 0.0, 0.0, 0.0, 0.0, 0.0, 0.0, 0.0, 0.0, 0.0, 0.0, 0.0, 0.0, 0.0, 0.0, 0.0, 0.0, 0.0, 0.0, 0.0, 0.0, 0.0, 0.0, 0.0, 0.0, 0.0, 0.0, 0.0, 0.0, 0.0, 0.0, 0.0, 0.0, 0.0, 0.0, 0.0, 0.0, 0.0, 0.0, 0.0, 0.0, 0.0, 0.0, 0.0, 0.0, 0.0, 0.0, 0.0, 0.0, 0.0, 0.0, 0.0, 0.0, 0.0, 0.0, 0.0, 0.0, 0.0, 0.0, 0.0, 0.0, 0.0, 0.0, 0.0, 0.0, 0.0, 0.0, 0.0, 0.0, 0.0, 0.0, 0.0, 0.0, 0.0, 0.0, 0.0, 0.0, 0.0, 0.0, 0.0, 0.0, 0.0, 0.0, 0.0, 0.0, 0.0, 0.0, 0.0, 0.0, 0.0, 0.0, 0.0, 0.0, 0.0, 0.0, 0.0, 0.0, 0.0, 0.0, 0.0, 0.0, 0.0, 0.0, 0.0, 0.0, 0.0, 0.0, 0.0, 0.0, 0.0, 0.0, 0.0, 0.0, 0.0, 0.0, 0.0, 0.0, 0.0, 0.0, 0.0, 0.0, 0.0, 0.0, 0.0, 0.0, 0.0, 0.0, 0.0, 0.0, 0.0, 0.0, 0.0, 0.0, 0.0, 0.0, 0.0, 0.0, 0.0, 0.0, 0.0, 0.0, 0.0, 0.0, 0.0, 0.0, 0.0, 0.0, 0.0, 0.0, 0.0, 0.0, 0.0, 0.0, 0.0, 0.0, 0.0, 0.0, 0.0, 0.0, 0.0, 0.0, 0.0, 0.0, 0.0, 0.0, 0.0, 0.0, 0.0, 0.0, 0.0, 0.0, 0.0, 0.0, 0.0, 0.0, 0.0, 0.0, 0.0, 0.0, 0.0, 0.0, 0.0, 0.0, 0.0, 0.0, 0.0, 0.0, 0.0, 0.0, 0.0, 0.0, 0.0, 0.0, 0.0, 0.0, 0.0, 0.0, 0.0, 0.0, 0.0, 0.0, 0.0, 0.0, 0.0, 0.0, 0.0, 0.0, 0.0, 0.0, 0.0, 0.0, 0.0, 0.0, 0.0, 0.0, 0.0, 0.0, 0.0, 0.0, 0.0, 0.0, 0.0, 0.0, 0.0, 0.0, 0.0, 0.0, 0.0, 0.0, 0.0, 0.0, 0.0, 0.0, 0.0, 0.0, 0.0, 0.0, 0.0, 0.0, 0.0, 0.0, 0.0, 0.0, 0.0, 0.0, 0.0, 0.0, 0.0, 0.0, 0.0, 0.0, 0.0, 0.0, 0.0, 0.0, 0.0, 0.0, 0.0, 0.0, 0.0, 0.0, 0.0, 0.0, 0.0, 0.0, 0.0, 0.0, 0.0, 0.0, 0.0, 0.0, 0.0, 0.0, 0.0, 0.0, 0.0, 0.0, 0.0, 0.0, 0.0, 0.0, 0.0, 0.0, 0.0, 0.0, 0.0, 0.0, 0.0, 0.0, 0.0, 0.0, 0.0, 0.0, 0.0, 0.0, 0.0, 0.0, 0.0, 0.0, 0.0, 0.0, 0.0, 0.0, 0.0, 0.0, 0.0, 0.0, 0.0, 0.0, 0.0, 0.0, 0.0, 0.0, 0.0, 0.0, 0.0, 0.0, 0.0, 0.0, 0.0, 0.0, 0.0, 0.0, 0.0, 0.0, 0.0, 0.0, 0.0, 0.0, 0.0, 0.0, 0.0, 0.0, 0.0, 0.0, 0.0, 0.0, 0.0, 0.0, 0.0, 0.0, 0.0, 0.0, 0.0, 0.0, 0.0, 0.0, 0.0, 0.0, 0.0, 0.0, 0.0, 0.0, 0.0, 0.0, 0.0, 0.0, 0.0, 0.0, 0.0, 0.0, 0.0, 0.0, 0.0, 0.0, 0.0, 0.0, 0.0, 0.0, 0.0, 0.0, 0.0, 0.0, 0.0, 0.0, 0.0, 0.0, 0.0, 0.0, 0.0, 0.0, 0.0, 0.0, 0.0, 0.0, 0.0, 0.0, 0.0, 0.0, 0.0, 0.0, 0.0, 0.0, 0.0, 0.0, 0.0, 0.0, 0.0, 0.0, 0.0, 0.0, 0.0, 0.0, 0.0, 0.0, 0.0, 0.0, 0.0, 0.0, 0.0, 0.0, 0.0, 0.0, 0.0, 0.0, 0.0, 0.0, 0.0, 0.0, 0.0, 0.0, 0.0, 0.0, 0.0, 0.0, 0.0, 0.0, 0.0, 0.0, 0.0, 0.0, 0.0, 0.0, 0.0, 0.0, 0.0, 0.0, 0.0, 0.0, 0.0, 0.0, 0.0, 0.0, 0.0, 0.0, 0.0, 0.0, 0.0, 0.0, 0.0, 0.0, 0.0, 0.0, 0.0, 0.0, 0.0, 0.0, 0.0, 0.0, 0.0, 0.0, 0.0, 0.0, 0.0, 0.0, 0.0, 0.0, 0.0, 0.0, 0.0, 0.0, 0.0, 0.0, 0.0, 0.0, 0.0, 0.0, 0.0, 0.0, 0.0, 0.0, 0.0, 0.0, 0.0, 0.0, 0.0, 0.0, 0.0, 0.0, 0.0, 0.0, 0.0, 0.0, 0.0, 0.0, 0.0, 0.0, 0.0, 0.0, 0.0, 0.0, 0.0, 0.0, 0.0, 0.0, 0.0, 0.0, 0.0, 0.0, 0.0, 0.0, 0.0, 0.0, 0.0, 0.0, 0.0, 0.0, 0.0, 0.0, 0.0, 0.0, 0.0, 0.0, 0.0, 0.0, 0.0, 0.0, 0.0, 0.0, 0.0, 0.0, 0.0, 0.0, 0.0, 0.0, 0.0, 0.0, 0.0, 0.0, 0.0, 0.0, 0.0, 0.0, 0.0, 0.0, 0.0, 0.0, 0.0, 0.0, 0.0, 0.0] -> [w480]
                i -> [w478]
                n138 = call "ReadSpectrum(SubVI).vi"("Continuous \nStrobe Delay"=w482, "Enter the \nInetegration Time"=w483) -> ("Spectrum Values"=w481:dbl[], "WL Values"=w484:dbl[], "Number of Spectrometers"=w485:i32)  [unwired: 7 in]
                n139 = Add(x=w481, y=w480) -> (x+y=w479:dbl[])
                "Number of time the OCEAN averaging loop has run -1" <- w478
              }
              "Number of Spectrometers" <- w474
              n140 = Divide(x=w457, y="Number of averages") -> (x/y=w456:dbl[])
              n141 = case shown="False" w469 {
                tunnel: w468 -> [_ w497]
                tunnel: w456 -> [w493 w496]
                tunnel: [w492 w495] -> w466
                tunnel: w465 -> [w494 _]
                frame False {
                  # "Matrix + int on i >3"
                  n142 = Build Array (concatenate)(w494, w493) -> (w492:dbl[][])
                }
                frame True {
                  # "WL + Int on =3"
                  n143 = Build Array(w497, w496) -> (w495:dbl[][])
                }
              }
              n144 = Bundle("WL Values"=w468, w456) -> (→"?":cluster{"WL Values":dbl[], dbl[]})  [unwired: 1 in]
              n145 = property on="Use autolab?" class="Bool (strict)"() -> ("Value"=w458:bool)  [unwired: 2 in, 2 out]
              n146 = case shown="True" w458 {
                tunnel: [SECenumctl."Apply potential" SECenumctl."Apply potential Autolab"] -> w459
                frame False {
                }
                frame True {
                }
              }
              n147 = case shown="False" w464 {
                tunnel: [0.0 1.0] -> w477
                tunnel: [1.0 ("Stop \npotential") 0.0 ("Stop \npotential")] -> w476
                frame False {
                }
                frame True {
                }
              }
            }
          }
          n148 = case shown="False" w209 {
            tunnel: w221 -> [w231 w233]
            tunnel: w219 -> [w230 w232]
            tunnel: [w229 w234] -> w208
            frame False {
              n149 = Greater Or Equal?(x=w231, y=w230) -> (x >= y?=w229:bool)
            }
            frame True {
              n150 = Less Or Equal?(x=w233, y=w232) -> (x <= y?=w234:bool)
            }
          }
        }
        n151 = Unbundle By Name(w158) -> ("Default\n potential"=w179:dbl)
        n152 = property on="Use autolab?" class="Bool (strict)"() -> ("Value"=w153:bool)  [unwired: 2 in, 2 out]
        n153 = Insert Into Array(array=w160, index=0, new element=0.0 ("new element/subarray")) -> (w169:dbl[])
        n154 = Transpose Matrix(1:w173) -> (0:w172:dbl[][])
        n155 = Bundle(w160, w164) -> (→"?":cluster{dbl[], dbl[]})  [unwired: 1 in]
        n156 = Reverse 1D Array(array=w169) -> (reversed array=w168:dbl[])
        n157 = property on="V (during measurment)" class="DigNum (strict)"("Value"=w179) -> ()  [unwired: 2 in, 2 out]
        n158 = case shown="True" w153 {
          tunnel: w179 -> [w187 w189]
          frame False {
            n159 = call "IV setpotential.vi"("value"=w187) -> ()  [unwired: 8 in, 3 out]
          }
          frame True {
            n160 = property on="Ei" class="Ref (strict)"() -> ("Value"=w188:refnum<k24>)  [unwired: 2 in, 2 out]
            n161 = property class="EI"(reference=w188, "Setpoint"=w189) -> ()  [unwired: 1 in, 2 out]
          }
        }
        n162 = Replace Array Subset(array=w172, new element=w168, index (row)=0 ("index")) -> (w157:dbl[][])  [unwired: 1 in]
        n163 = Bundle By Name(cluster=w158, "Spectrum"=w172, "Current array"=w164, "Potential array"=w160) -> (w159:T11)
        n164 = Build Array(w160, w164) -> (w171:dbl[][])
        n165 = disable-structure shown="Enabled" {
          disable-tunnel: w157 -> [w205 _]
          disable-tunnel: w158 -> [w204 _]
          frame Enabled {
            n166 = call "WriteSEC.vi"("Init cluster"=w204, "Array"=w205) -> ()  [unwired: 10 in]
          }
          frame Disabled {
          }
        }
        n167 = Transpose Matrix(1:w171) -> (0:w170:dbl[][])
        n168 = disable-structure shown="Enabled" {
          disable-tunnel: w170 -> [w203 _]
          disable-tunnel: w159 -> [w202 _]
          frame Enabled {
            n169 = call "Write_JV.vi"("Init cluster"=w202, "Array"=w203) -> ()  [unwired: 10 in]
          }
          frame Disabled {
          }
        }
      }
      frame "Exit" {
        w501 = TRUE  # Stop Loop?
        w504 = State."Exit"  # (Value Not Used)
        # "Switch cell on/off"
        # "Diconnect device and close Ivium remdriver"
        # "Disconnect Ivium device (when connected)\nbefore terminating this VI"
        # "Exit - Exit the application."
        n170 = property on="Shut down sequence run?" class="Bool (strict)"("Value"=FALSE ("Shut down sequence run?")) -> ()  [unwired: 2 in, 2 out]
        n171 = property on="PotentialOverload" class="Bool (strict)"("Value"=FALSE ("PotentialOverload")) -> ()  [unwired: 2 in, 2 out]
        n172 = property on="T reached?" class="Bool (strict)"("Value"=FALSE ("T reached?")) -> ()  [unwired: 2 in, 2 out]
        n173 = property on="Use autolab?" class="Bool (strict)"() -> ("Value"=w502:bool)  [unwired: 2 in, 2 out]
        n174 = case shown="True" w502 {
          tunnel: [w516 w534] -> w508
          tunnel: w507 -> [w513 w529]
          tunnel: [w511 0 ("devconnect")] -> w506
          frame False {
            w509 = FALSE ("Shut down sequence run?")
            # "This re-initialises a display for the iDus camera"
            # "On"
            # "Close Ivium Driver"
            n175 = To Long Integer(number=0) -> (32bit integer=w515:i32)
            n176 = call "IV setcellon.vi"("error in (no error)"=w513, "cellon"=w515) -> ("error out"=w512:errorcluster)  [unwired: 7 in, 2 out]
            n177 = call "IV getdevicestatus.vi"("error in (no error)"=w512) -> ("error out"=w517:errorcluster, "return type"=w518:i32)  [unwired: 9 in]
            n178 = Greater Than 0?(x=w518) -> (x > 0?=w510:bool)
            n179 = case shown="False" w510 {
              tunnel: [w521 w523] -> w519
              tunnel: w517 -> [w521 _]
              tunnel: [0 ("devconnect") w522] -> w511
              frame False {
              }
              frame True {
                w522 = 0 ("devconnect")
                n180 = call "IV connect.vi"("devconnect"=w522) -> ("error out"=w523:errorcluster)  [unwired: 8 in, 2 out]
              }
            }
            n181 = property on="Shut down sequence run?" class="Bool (strict)"("Value"=w509) -> ()  [unwired: 2 in, 2 out]
            n182 = property on="Return detector \nto room T?" class="Bool (strict)"("Value"=w509) -> ()  [unwired: 2 in, 2 out]
            n183 = call "IV close.vi"("error in (no error)"=w519) -> ("error out"=w516:errorcluster)  [unwired: 9 in, 1 out]
          }
          frame True {
            w528 = 0 items=["Off", "On"] ("CellOnOff")
            n184 = property on="Ei" class="Ref (strict)"() -> ("Value"=w527:refnum<k24>)  [unwired: 2 in, 2 out]
            n185 = property class="EI"(reference=w527, error in=w529, "CellOnOff"=w528) -> (error out=w526:errorcluster)  [unwired: 1 out]
            n186 = property on="ManualCellSwitch" class="Bool (strict)"("Value"=FALSE ("ManualCellSwitch")) -> ()  [unwired: 2 in, 2 out]
            n187 = property on="Cell on?" class="Bool (strict)"("Value"=FALSE ("Cell")) -> ()  [unwired: 2 in, 2 out]
            n188 = property on="instrument" class="Ref (strict)"(error in=w526) -> (error out=w532:errorcluster, "Value"=w533:refnum<k24>)  [unwired: 1 in, 1 out]
            n189 = property on="Autolab Connected?" class="Bool (strict)"("Value"=FALSE ("IsConnected")) -> ()  [unwired: 2 in, 2 out]
            n190 = invoke class="Instrument" method="Disconnect"(reference=w533, error in=w532) -> (error out=w534:errorcluster)  [unwired: 1 in, 2 out]
          }
        }
        n191 = property on="V2 applied?" class="Bool (strict)"("Value"=FALSE ("V2 applied")) -> ()  [unwired: 2 in, 2 out]
      }
      frame "Run OSPEC" {
        n192 = property on="Use autolab?" class="Bool (strict)"() -> ("Value"=w536:bool)  [unwired: 2 in, 2 out]
        n193 = case shown="True" w536 {
          tunnel: w543 -> [w549 w557]
          tunnel: [w548 w557] -> w542
          frame False {
            # "Get cell status"
            # "Get Device Status"
            # "Direct Mode"
            n194 = call "IV getdevicestatus.vi"() -> ("return type"=w552:i32)  [unwired: 10 in, 1 out]
            n195 = Increment(x=w552) -> (x+1=w551:i32)
            n196 = case shown="0, Default" w551 {
              tunnel: ["no IviumSoft" "device not connected" "device available_idle" "device available_busy"] -> w550
              frame 0, Default {
              }
              frame 1 {
              }
              frame 2 {
              }
              frame 3 {
              }
            }
            n197 = Bundle By Name(cluster=w549, "Status"=w550) -> (w548:T11)
          }
          frame True {
          }
        }
        n198 = while {
          shift-right: [w558] -> w540
          shift-left: w541 -> [w563]
          shift-right: [w559] -> w539
          shift-left: w542 -> [w565]
          shift-right: [w562] -> _
          shift-left: OSSPEC."Apply V1" -> [w564]
          i -> [w561]
          stop <- w560 stop-if-true
          n199 = case shown="\"Read current and spectrum\"" w564 {
            tunnel: w565 -> [w569 w956 w1471 w1495 w1557 w1620]
            tunnel: w563 -> [w568 w972 w1475 w1494 w1567 w1648]
            tunnel: [OSSPEC."End measurment" w988 OSSPEC."Read Potential and spectrum" OSSPEC."Read current and spectrum" OSSPEC."Read current and spectrum" OSSPEC."End measurment"] -> w562
            tunnel: [w574 w971 w1474 w1490 w1558 w1646] -> w558
            tunnel: [w575 w979 w1471 w1491 w1557 w1620] -> w559
            tunnel: w561 -> [_ _ _ _ _ _]
            tunnel: [FALSE FALSE FALSE FALSE FALSE w1647] -> w560
            frame "Read Potential and spectrum", Default {
              n200 = property on="Use autolab?" class="Bool (strict)"() -> ("Value"=w566:bool)  [unwired: 2 in, 2 out]
              n201 = disable-structure shown="Enabled" {
                disable-tunnel: w568 -> [w590 _]
                disable-tunnel: [w589 _] -> w567
                disable-tunnel: w566 -> [w588 _]
                frame Enabled {
                  n202 = case shown="True" w588 {
                    tunnel: w590 -> [w592 w604]
                    tunnel: [w591 w602] -> w589
                    frame False {
                      n203 = flat-sequence {
                        tunnel: w592 -> [w595]
                        tunnel: [w595] -> w593
                        tunnel: [w596] -> w591
                        tunnel: w593 -> [w597]
                        frame #0 {
                          n204 = Wait (ms)(milliseconds to wait=u32 50) -> ()  [unwired: 1 out]
                        }
                        frame #1 {
                          n205 = To Long Integer(number=T17."IStat4EL" ("Configuration")) -> (32bit integer=w599:i32)
                          n206 = call "IV setconnectionmode.vi"("error in (no error)"=w597, "value"=w599) -> ("error out"=w596:errorcluster)  [unwired: 7 in, 2 out]
                        }
                      }
                    }
                    frame True {
                      w600 = 0 items=["Off", "On"] ("CellOnOff")
                      w605 = -6 items=["CR07_1A"=0, "CR06_10A"=1, "CR01_100A"=2, "CR00_1000A"=3, "CR05_20A"=20, "CR04_40A"=40, "CR03_50A"=60, "CR02_80A"=80, "CR19_1pA"=-12, "CR18_10pA"=-11, "CR17_100pA"=-10, "CR16_1nA"=-9, "CR15_10nA"=-8, "CR14_100nA"=-7, "CR13_1uA"=-6, "CR12_10uA"=-5, "CR11_100uA"=-4, "CR10_1mA"=-3, "CR09_10mA"=-2, "CR08_100mA"=-1] ("CurrentRange")
                      w606 = 0 items=["Potentiostatic", "Galvanostatic"] ("Mode")
                      n207 = property on="Ei" class="Ref (strict)"() -> ("Value"=w601:refnum<k24>)  [unwired: 2 in, 2 out]
                      n208 = property class="EI"(reference=w601, error in=w604, "CurrentRange"=w605) -> (error out=w603:errorcluster)  [unwired: 1 out]
                      n209 = property class="EI"(reference=w601, error in=w603, "Mode"=w606, "CellOnOff"=w600) -> (error out=w602:errorcluster)  [unwired: 1 out]
                    }
                  }
                }
                frame Disabled {
                }
              }
              n210 = Unbundle By Name(w569) -> ("Spectrum"=w577:dbl[][])
              n211 = Unbundle By Name(w569) -> ("Time for spectrum measurment"=w576:i32[], "Start time"=w579:i32)
              n212 = Unbundle By Name(w569) -> ("Potential array"=w572:dbl[])
              n213 = property on="Use iDus?" class="Bool (strict)"() -> ("Value"=w570:bool)  [unwired: 2 in, 2 out]
              n214 = Unbundle By Name(w569) -> ("Time for E measurment"=w571:i32[], "Start time"=w578:i32)
              n215 = while {
                shift-right: [w838] -> _
                shift-left: w569 -> [w839]
                shift-right: [w830] -> _
                shift-left: OSPEC-enum."Wait" -> [w840]
                shift-right: [w837] -> w582
                shift-left: w571 -> [w836]
                shift-right: [w831] -> w581
                shift-left: w572 -> [w834]
                shift-right: [w833] -> _
                shift-left: w578 -> [w832]
                shift-right: [w828] -> w574
                shift-left: w567 -> [w829]
                i -> [w835]
                stop <- w825 stop-if-true
                n216 = case shown="\"Read\", Default" w840 {
                  tunnel: w839 -> [w848 w859 w950]
                  tunnel: [w848 w859 w950] -> w838
                  tunnel: [w847 FALSE FALSE] -> w827
                  tunnel: [w852 w863 w948] -> w837
                  tunnel: w836 -> [w852 w864 w948]
                  tunnel: w835 -> [_ w868 _]
                  tunnel: [w850 w867 w945] -> w831
                  tunnel: w834 -> [w850 w866 w945]
                  tunnel: [w843 w860 w947] -> w833
                  tunnel: w832 -> [w843 _ w947]
                  tunnel: [OSPEC-enum."Wait" OSPEC-enum."Check exit" OSPEC-enum."Read"] -> w830
                  tunnel: w829 -> [w849 w856 w944]
                  tunnel: [w849 w855 w944] -> w828
                  frame "Check exit" {
                    n217 = Unbundle By Name(w848) -> ("V off time"=w845:dbl)
                    n218 = Multiply(x=w845, y=1000.0) -> (x*y=w846:dbl)
                    n219 = Greater Or Equal?(x=w843, y=w846) -> (x >= y?=w847:bool)
                  }
                  frame "Read", Default {
                    # "Building a 1d matrix of potentials and times"
                    n220 = property on="Use autolab?" class="Bool (strict)"() -> ("Value"=w853:bool)  [unwired: 2 in, 2 out]
                    n221 = case shown="True" w853 {
                      tunnel: [w871 w874] -> w857
                      tunnel: w856 -> [w870 w872]
                      tunnel: [w869 w873] -> w855
                      frame False {
                        n222 = call "IV getpotential.vi"("error in (no error)"=w870) -> ("error out"=w869:errorcluster, "value out"=w871:dbl)  [unwired: 8 in, 1 out]
                      }
                      frame True {
                        n223 = disable-structure shown="Enabled" {
                          disable-tunnel: [w879 _ w925] -> w874
                          disable-tunnel: [w878 _ w927] -> w873
                          disable-tunnel: w872 -> [w876 _ w935]
                          frame Disabled {
                            n224 = property on="Ei" class="Ref (strict)"() -> ("Value"=w877:refnum<k24>)  [unwired: 2 in, 2 out]
                            n225 = disable-structure shown="Enabled" {
                              disable-tunnel: w877 -> [w887 _]
                              disable-tunnel: w876 -> [w883 w888]
                              disable-tunnel: [w882 w888] -> w875
                              frame Disabled {
                                w884 = -4 items=["CR07_1A"=0, "CR06_10A"=1, "CR01_100A"=2, "CR00_1000A"=3, "CR05_20A"=20, "CR04_40A"=40, "CR03_50A"=60, "CR02_80A"=80, "CR19_1pA"=-12, "CR18_10pA"=-11, "CR17_100pA"=-10, "CR16_1nA"=-9, "CR15_10nA"=-8, "CR14_100nA"=-7, "CR13_1uA"=-6, "CR12_10uA"=-5, "CR11_100uA"=-4, "CR10_1mA"=-3, "CR09_10mA"=-2, "CR08_100mA"=-1] ("CurrentRange")
                                w886 = 1 items=["Potentiostatic", "Galvanostatic"] ("Mode")
                                n226 = property class="EI"(reference=w887, error in=w883, "Mode"=w886, "Setpoint"=0.0, "CurrentRange"=w884) -> (error out=w882:errorcluster)  [unwired: 1 out]
                              }
                              frame Enabled {
                              }
                            }
                            n227 = property class="EI"(reference=w877, error in=w875) -> (error out=w878:errorcluster, "Current"=w880:dbl, "Potential"=w879:dbl)  [unwired: 1 out]
                            n228 = disable-structure shown="Enabled" {
                              disable-tunnel: w880 -> [w881 _]
                              frame Disabled {
                                "OCP I (close to 0)" <- w881
                              }
                              frame Enabled {
                              }
                            }
                          }
                          frame Disabled {
                            n229 = property on="Property Node" class="Ref (strict)"() -> ("Value"=w890:refnum<k24>)  [unwired: 2 in, 2 out]
                            n230 = disable-structure shown="Disabled" {
                              disable-tunnel: _ -> [w916 _]
                              disable-tunnel: [w915 _] -> _
                              disable-tunnel: _ -> [w912 _]
                              disable-tunnel: w890 -> [w911 _]
                              frame Disabled {
                                w909 = 2 items=["UltraHigh_Speed", "High_Speed", "High_Stability"] ("Bandwidth")
                                w914 = 1 items=["Off", "On"] ("CellOnOff")
                                w910 = 0 items=["Potentiostatic", "Galvanostatic"] ("Mode")
                                n231 = property on="Property Node" class="Ring (strict)"() -> ("Value"=w913:i32)  [unwired: 2 in, 2 out]
                                n232 = property class="EI"(reference=w911, error in=w912, "Bandwidth"=w909, "CellOnOff"=w914, "CurrentRange"=w913, "Mode"=w910, "Setpoint"=w916) -> (error out=w915:errorcluster)  [unwired: 1 out]
                                n233 = property on="Property Node" class="Ref (strict)"(error in=w915) -> (error out=w908:errorcluster, "Value"=w905:refnum<k24>)  [unwired: 1 in, 1 out]
                                n234 = property class="EI"(reference=w911, error in=w915) -> (error out=w906:errorcluster, "EiStatusSupportedFor"=w907:string[])  [unwired: 1 out]
                                n235 = invoke class="Sampler" method="Sample"(reference=w905, error in=w908) -> ()  [unwired: 1 in, 3 out]
                                n236 = property on="Property Node" class="Arr (strict)"(error in=w906, "Value"=w907) -> ()  [unwired: 1 in, 2 out]
                              }
                              frame Enabled {
                              }
                            }
                            n237 = property class="EI"(reference=w890) -> (error in=w892:errorcluster, error out=w891:errorcluster, "Setpoint"=w889:dbl)  [unwired: 1 out]
                            n238 = property class="EI" props=["Bandwidth", "CurrentRange", "Mode", "Setpoint", "Current", "Potential"](reference=w890, error in=w891) -> (error out=w893:errorcluster, "Bandwidth"=w904:i32, "CurrentRange"=w903:i32, "Mode"=w902:i32, "Current"=w896:dbl, "Potential"=w895:dbl)  [unwired: 2 out]
                            n239 = property on="Property Node" class="Ring (strict)"("Value"=w904) -> ()  [unwired: 2 in, 2 out]
                            n240 = property on="Property Node" class="Ring (strict)"("Value"=w903) -> ()  [unwired: 2 in, 2 out]
                            n241 = property on="Property Node" class="Ring (strict)"("Value"=w902) -> ()  [unwired: 2 in, 2 out]
                            n242 = flat-sequence {
                              tunnel: [w920] -> w901
                              tunnel: w896 -> [w919]
                              tunnel: w895 -> [w918]
                              tunnel: [w917] -> w894
                              tunnel: w893 -> [w917]
                              frame #0 {
                                n243 = call "Range_selector.vi"("potential"=w918, "current"=w919) -> ("range integer"=w920:i32)  [unwired: 9 in]
                              }
                            }
                            n244 = property class="EI"(reference=w890, error in=w894) -> (error out=w900:errorcluster, "Current"=→"Current PD 2":dbl, "Potential"=→"POtential PD 2":dbl)  [unwired: 1 out]
                            n245 = property class="EI"(reference=w890, error in=w900, "CurrentRange"=w901) -> (error out=w899:errorcluster)  [unwired: 1 out]
                          }
                          frame Enabled {
                            w922 = -9 items=["CR07_1A"=0, "CR06_10A"=1, "CR01_100A"=2, "CR00_1000A"=3, "CR05_20A"=20, "CR04_40A"=40, "CR03_50A"=60, "CR02_80A"=80, "CR19_1pA"=-12, "CR18_10pA"=-11, "CR17_100pA"=-10, "CR16_1nA"=-9, "CR15_10nA"=-8, "CR14_100nA"=-7, "CR13_1uA"=-6, "CR12_10uA"=-5, "CR11_100uA"=-4, "CR10_1mA"=-3, "CR09_10mA"=-2, "CR08_100mA"=-1] ("CurrentRange")
                            w932 = -9 items=["CR07_1A"=0, "CR06_10A"=1, "CR01_100A"=2, "CR00_1000A"=3, "CR05_20A"=20, "CR04_40A"=40, "CR03_50A"=60, "CR02_80A"=80, "CR19_1pA"=-12, "CR18_10pA"=-11, "CR17_100pA"=-10, "CR16_1nA"=-9, "CR15_10nA"=-8, "CR14_100nA"=-7, "CR13_1uA"=-6, "CR12_10uA"=-5, "CR11_100uA"=-4, "CR10_1mA"=-3, "CR09_10mA"=-2, "CR08_100mA"=-1] ("CurrentRange")
                            w936 = 0 items=["Off", "On"] ("CellOnOff")
                            w937 = 1 items=["UltraHigh_Speed", "High_Speed", "High_Stability"] ("Bandwidth")
                            w938 = 1 items=["Potentiostatic", "Galvanostatic"] ("Mode")
                            w942 = 1 items=["Potentiostatic", "Galvanostatic"] ("Mode")
                            w924 = 0 items=["Off", "On"] ("CellOnOff")
                            w943 = 1 items=["UltraHigh_Speed", "High_Speed", "High_Stability"] ("Bandwidth")
                            n246 = property on="Ei" class="Ref (strict)"() -> ("Value"=w934:refnum<k24>)  [unwired: 2 in, 2 out]
                            n247 = property on="Sampler 2" class="Ref (strict)"() -> ("Value"=w933:refnum<k24>)  [unwired: 2 in, 2 out]
                            n248 = call "EI (A).vi"("Sampler"=w933, "Ei"=w934, "CellOnOff"=w924, "Setpoint"=0.0, "Bandwidth"=w943, "CurrentRange"=w932, "Mode"=w942, "error in (no error)"=w935, "Disable Sampler"=FALSE) -> ("Cell"=w931:bool, "PotentialOverload"=w930:bool, "Setpoint"=→"Setpoint":dbl, "error out"=w928:errorcluster)  [unwired: 5 in, 10 out]
                            n249 = property on="PotentialOverload" class="Bool (strict)"("Value"=w930) -> ()  [unwired: 2 in, 2 out]
                            n250 = property on="Cell on?" class="Bool (strict)"("Value"=w931) -> ()  [unwired: 2 in, 2 out]
                            n251 = call "Sampler.vi"("error in (no error)"=w935, "Sampler"=w933) -> ("error out"=w940:errorcluster)  [unwired: 7 in, 2 out]
                            n252 = Merge Errors(w940, w928) -> (w941:errorcluster)
                            n253 = call "EI (A).vi"("Sampler"=w933, "Ei"=w934, "CellOnOff"=w936, "Bandwidth"=w937, "CurrentRange"=w922, "Mode"=w938, "error in (no error)"=w941, "Disable Sampler"=FALSE) -> ("Potential"=w925:dbl, "Current"=w926:dbl, "error out"=w927:errorcluster)  [unwired: 6 in, 11 out]
                            "Potential  During PD" <- w925
                            n254 = property on="current" class="DigNum (strict)"("Value"=w926) -> ()  [unwired: 2 in, 2 out]
                            n255 = property on="Voltage" class="DigNum (strict)"("Value"=w925) -> ()  [unwired: 2 in, 2 out]
                          }
                        }
                      }
                    }
                    "OCP" <- w857
                    n256 = Unbundle By Name(w859) -> ("Start time"=w858:i32)
                    n257 = Tick Count (ms)() -> (millisecond timer value=w854:u32)
                    n258 = Subtract(x=w854, y=w858) -> (x-y=w860:u32)
                    n259 = Equal?(x=1, y=w868) -> ()  [unwired: 1 out]
                    n260 = Build Array (concatenate)(w864, w860) -> (w863:u32[])
                    n261 = Build Array (concatenate)(w866, w857) -> (w867:dbl[])
                  }
                  frame "Wait" {
                    n262 = Unbundle By Name(w950) -> ("Sample rate"=w951:dbl)
                    n263 = Multiply(x=w951, y=1000.0) -> (x*y=w953:dbl)
                    n264 = Wait (ms)(milliseconds to wait=w953) -> ()  [unwired: 1 out]
                  }
                }
                n265 = property on="Use iDus?" class="Bool (strict)"() -> ("Value"=w824:bool)  [unwired: 2 in, 2 out]
                n266 = case shown="False" w824 {
                  tunnel: [TRUE ("Value") w842] -> w826
                  frame False {
                  }
                  frame True {
                    n267 = property on="IDus not in read loop? (kinetic)" class="Bool (strict)"() -> ("Value"=w842:bool)  [unwired: 2 in, 2 out]
                  }
                }
                n268 = And(x=w826, y=w827) -> (x .and. y?=w825:bool)
              }
              n269 = case shown="False" w570 {
                tunnel: [w620 w699] -> w584
                tunnel: [w619 w700] -> w583
                tunnel: w579 -> [w618 w706]
                tunnel: w577 -> [w617 w704]
                tunnel: w576 -> [w616 w702]
                tunnel: [w615 w701] -> w573
                tunnel: w569 -> [w614 w705]
                frame False {
                  n270 = disable-structure shown="Enabled" {
                    disable-tunnel: w614 -> [w632 _]
                    disable-tunnel: [w629 w633] -> w613
                    disable-tunnel: [w628 w635] -> w612
                    disable-tunnel: [w627 w634] -> w611
                    frame Disabled {
                      n271 = Unbundle By Name(w632) -> ("Continous strobe delay"=w630:i32, "Integration time"=w631:i32)
                      n272 = call "OSPEC-Open-Ocean.vi"("Integration Time"=w630, "delay"=w631) -> ("WL Values"=w629:dbl[], "Wrapper Out"=w627:u32, "ContinuousStrobe Out"=w628:u32)  [unwired: 7 in]
                    }
                    frame Enabled {
                      n273 = property on="WL Values" class="Arr (strict)"() -> ("Value"=w633:dbl[])  [unwired: 2 in, 2 out]
                      n274 = property on="ContinuousStrobe Out" class="DigNum (strict)"() -> ("Value"=w635:u32)  [unwired: 2 in, 2 out]
                      n275 = property on="Wrapper Out" class="DigNum (strict)"() -> ("Value"=w634:u32)  [unwired: 2 in, 2 out]
                    }
                  }
                  n276 = while {
                    shift-right: [w650] -> _
                    shift-left: w614 -> [w651]
                    shift-right: [w643] -> _
                    shift-left: OSPEC-enum."Read" -> [w652]
                    shift-right: [w648] -> w619
                    shift-left: w616 -> [w647]
                    shift-right: [w642] -> w615
                    shift-left: w617 -> [w646]
                    shift-right: [w645] -> w620
                    shift-left: w618 -> [w639]
                    tunnel: w611 -> [w641]
                    tunnel: [w640] -> w608
                    tunnel: w613 -> [w638]
                    tunnel: [w637] -> w607
                    tunnel: w612 -> [w636]
                    i -> [w644]
                    stop <- w649 stop-if-true
                    n277 = case shown="\"Read\", Default" w652 {
                      tunnel: w651 -> [w662 w674 w693]
                      tunnel: [w662 w674 w693] -> w650
                      tunnel: [w661 FALSE FALSE] -> w649
                      tunnel: [w664 w680 w691] -> w648
                      tunnel: w647 -> [w664 w679 w691]
                      tunnel: w644 -> [_ _ _]
                      tunnel: [w660 w675 w687] -> w642
                      tunnel: w646 -> [w660 w678 w687]
                      tunnel: [w653 w671 w684] -> w645
                      tunnel: w639 -> [w653 _ w684]
                      tunnel: [OSPEC-enum."Wait" OSPEC-enum."Check exit" OSPEC-enum."Read"] -> w643
                      tunnel: w641 -> [w658 w665 w688]
                      tunnel: [w659 w670 w689] -> _
                      tunnel: w638 -> [w659 w670 w689]
                      tunnel: [w658 w665 w688] -> w640
                      tunnel: [w655 w668 w682] -> w637
                      tunnel: w636 -> [w655 w668 w682]
                      frame "Check exit" {
                        n278 = Unbundle By Name(w662) -> ("V off time"=w657:dbl)
                        n279 = Multiply(x=w657, y=1000.0) -> (x*y=w654:dbl)
                        n280 = Greater Or Equal?(x=w653, y=w654) -> (x >= y?=w661:bool)
                      }
                      frame "Read", Default {
                        # "Continue 2d matrix of specta"
                        # "Continue to add times to this"
                        n281 = Tick Count (ms)() -> (millisecond timer value=w672:u32)
                        n282 = call "Wrapper_getSpectrum.vi"("Index"=0, "Wrapper"=w665) -> ("Spectrum Values"=w667:dbl[])  [unwired: 1 out]
                        n283 = Unbundle By Name(w674) -> ("Start time"=w673:i32)
                        n284 = Subtract(x=w672, y=w673) -> (x-y=w671:u32)
                        "Time during PD" <- w671
                        n285 = Bundle("Value"=w670, "Spectrum Values"=w667) -> (→"?":cluster{"Value":dbl[], "Spectrum Values":dbl[]})  [unwired: 1 in]
                        n286 = Build Array (concatenate)(w679, w671) -> (w680:u32[])
                        n287 = Build Array (concatenate)(w678, w667) -> (w675:dbl[][])
                      }
                      frame "Wait" {
                        n288 = Unbundle By Name(w693) -> ("Sample rate"=w694:dbl)
                        n289 = Multiply(x=1000.0, y="Slow sample time (s)") -> (x*y=w683:dbl)
                        n290 = Greater?(x=w684, y=w683) -> (0:w681:bool)
                        n291 = case shown="False" w681 {
                          tunnel: w694 -> [w695 _]
                          frame False {
                            n292 = Multiply(x=w695, y=1000.0) -> (x*y=w697:dbl)
                            n293 = Wait (ms)(milliseconds to wait=w697) -> ()  [unwired: 1 out]
                          }
                          frame True {
                            # "slow down read to measure slow decays\nwithout oversampling"
                            n294 = Wait (ms)(milliseconds to wait=u32 500) -> ()  [unwired: 1 out]
                          }
                        }
                      }
                    }
                  }
                  n295 = flat-sequence {
                    tunnel: [w624] -> w610
                    tunnel: [w623] -> w609
                    tunnel: w607 -> [w623]
                    tunnel: w608 -> [w622]
                    tunnel: w610 -> [w626]
                    tunnel: w609 -> [w625]
                    frame #0 {
                      # "Close spectrometers"
                      n296 = call "Wrapper_closeAllSpectrometers.vi"("Wrapper In"=w622) -> ("Wrapper Out"=w624:u32)
                    }
                    frame #1 {
                      # "Destroy \nwrapper \nand strobe"
                      n297 = call "ContinuousStrobe_Destroy.vi"("ContinuousStrobe"=w625) -> ()
                      n298 = call "Wrapper_Destroy.vi"("Wrapper"=w626) -> ()
                    }
                  }
                }
                frame True {
                  n299 = while {
                    shift-right: [w716] -> w699
                    shift-left: w706 -> [w717]
                    shift-right: [w709] -> _
                    shift-left: OSPEC-enum."Wait" -> [w718]
                    shift-right: [w715] -> w700
                    shift-left: w702 -> [w714]
                    shift-right: [w708] -> w701
                    shift-left: w704 -> [w713]
                    shift-right: [w712] -> _
                    shift-left: w705 -> [w711]
                    i -> [w710]
                    stop <- w707 stop-if-true
                    n300 = case shown="\"Wait\"" w718 {
                      tunnel: w717 -> [w720 _ w821]
                      tunnel: [w720 w729 w821] -> w716
                      tunnel: [w726 FALSE FALSE] -> w707
                      tunnel: [w728 w733 w819] -> w715
                      tunnel: w714 -> [w728 w737 w819]
                      tunnel: w710 -> [_ w740 _]
                      tunnel: w713 -> [w721 w736 w815]
                      tunnel: [w727 w731 w817] -> w712
                      tunnel: w711 -> [w727 w731 w817]
                      tunnel: [OSPEC-enum."Wait" OSPEC-enum."Check exit" OSPEC-enum."Read"] -> w709
                      tunnel: [w721 w734 w815] -> w708
                      frame "Check exit" {
                        n301 = Unbundle By Name(w727) -> ("V off time"=w722:dbl)
                        n302 = Multiply(x=w722, y=1000.0) -> (x*y=w723:dbl)
                        n303 = Greater Or Equal?(x=w720, y=w723) -> (x >= y?=w726:bool)
                      }
                      frame "Read", Default {
                        n304 = Unbundle By Name(w731) -> ("Start time"=w730:i32)
                        n305 = property on="Number of scans in kinetic cycle" class="DigNum (strict)"() -> ("Value"=w732:i32)  [unwired: 2 in, 2 out]
                        n306 = Tick Count (ms)() -> (millisecond timer value=w738:u32)
                        n307 = call "GetDetector.vi"() -> ("xpixels"=w739:i32)  [unwired: 4 in, 3 out]
                        n308 = Subtract(x=w738, y=w730) -> (x-y=w729:u32)
                        n309 = Equal?(x=w740, y=1.0) -> (x = y?=w735:bool)
                        n310 = stacked-sequence {
                          seq-local: [_ _ _ _ _ _ _ _ _ _ w774 _] -> [_ _ _ _ _ _ _ _ _ _ _ w794]
                          seq-local: [_ _ _ _ _ _ _ _ w759 _ _ _] -> [_ _ _ _ _ _ _ _ _ _ _ w792]
                          seq-local: [_ _ _ _ _ _ _ _ _ _ w773 _] -> [_ _ _ _ _ _ _ _ _ _ _ w793]
                          tunnel: [_ _ _ _ _ _ _ _ _ _ _ w787] -> w734
                          tunnel: [_ _ _ _ _ _ _ _ _ _ _ w788] -> w733
                          tunnel: w732 -> [_ _ _ _ _ w752 _ _ _ _ _ w786]
                          tunnel: w729 -> [_ _ _ _ _ _ _ _ _ _ _ w789]
                          tunnel: w729 -> [_ _ _ _ _ _ _ _ _ _ _ _]
                          tunnel: w739 -> [_ w745 _ _ _ _ _ _ _ _ _ _]
                          tunnel: w730 -> [_ _ _ _ _ _ _ _ w758 _ w772 _]
                          tunnel: w737 -> [_ _ _ _ _ _ _ _ _ _ _ w785]
                          tunnel: w736 -> [_ _ _ _ _ _ _ _ _ _ _ w784]
                          tunnel: w735 -> [_ _ _ _ _ _ _ _ _ _ _ w783]
                          frame #0 {
                            w744 = u16 3  # AcquisitionMode
                            n311 = call "SetAcquisitionMode.vi"("mode"=w744) -> ()  [unwired: 1 in, 2 out]
                          }
                          frame #1 {
                            w746 = u16 0  # ReadMode
                            n312 = property on="xpixels" class="DigNum (strict)"("Value"=w745) -> ()  [unwired: 2 in, 2 out]
                            n313 = call "SetReadMode.vi"("mode"=w746) -> ()  [unwired: 1 in, 2 out]
                          }
                          frame #2 {
                            n314 = call "SetTriggerMode.vi"("mode"=TriggerMode_mode_typedef."Internal") -> ()  [unwired: 1 in, 2 out]
                          }
                          frame #3 {
                            n315 = property on="Exposure time (s)" class="DigNum (strict)"() -> ("Value"=w748:dbl)  [unwired: 2 in, 2 out]
                            n316 = call "SetExposureTime.vi"("time"=w748) -> ()  [unwired: 1 in, 2 out]
                          }
                          frame #4 {
                            n317 = call "GetNumberVSSpeeds.vi"() -> ("number"=w751:i32)  [unwired: 3 in, 2 out]
                            n318 = Subtract(x=w751, y=1) -> (x-y=w749:i32)
                            n319 = call "SetVSSpeed.vi"("index"=w749) -> ()  [unwired: 1 in, 2 out]
                          }
                          frame #5 {
                            n320 = call "SetNumberKinetics.vi"("number"=w752) -> ()  [unwired: 1 in, 2 out]
                          }
                          frame #6 {
                            w755 = 0  # Auto Shutter
                            n321 = property on="Shutter open and close time" class="DigNum (strict)"() -> ("Value"=w753:i32)  [unwired: 2 in, 2 out]
                            n322 = property on="Shutter opens on TTL" class="Enum (strict)"() -> ("Value"=w754:T9)  [unwired: 2 in, 2 out]
                            n323 = call "SetShutter.vi"("type"=w754, "mode"=w755, "closingtime"=w753, "openingtime"=w753) -> ()  [unwired: 10 in, 2 out]
                          }
                          frame #7 {
                            # "Meybe delete the exposure time insupt here"
                            n324 = property on="Exposure time (s)" class="DigNum (strict)"() -> ("Value"=w757:dbl)  [unwired: 2 in, 2 out]
                            n325 = call "GetAcquisitionTimings.vi"("exposure input"=w757) -> ("exposure"=w756:sgl)  [unwired: 10 in, 4 out]
                            n326 = property on="Calculated exposure time" class="DigNum (strict)"("Value"=w756) -> ()  [unwired: 2 in, 2 out]
                          }
                          frame #8 {
                            n327 = flat-sequence {
                              tunnel: [w760] -> w759
                              tunnel: w758 -> [w761]
                              frame #0 {
                                n328 = Tick Count (ms)() -> (millisecond timer value=w762:u32)
                                n329 = Subtract(x=w762, y=w761) -> (x-y=w760:u32)
                                n330 = property on="Time before the start of current aquisition (ms)" class="DigNum (strict)"("Value"=w760) -> ()  [unwired: 2 in, 2 out]
                              }
                              frame #1 {
                                n331 = call "StartAcquisition.vi"() -> ("DLL error code"=w763:u32)  [unwired: 2 in, 1 out]
                                n332 = property on="Start Aquisition return code" class="DigNum (strict)"("Value"=w763) -> ()  [unwired: 2 in, 2 out]
                              }
                            }
                          }
                          frame #9 {
                            n333 = while {
                              stop <- w767 continue-if-true
                              w768 = u16 72  # DRV ACQUIRING
                              n334 = call "GetStatus.vi"() -> ("DLL error code"=w765:u32, "status"=w766:T18)  [unwired: 3 in, 1 out]
                              n335 = property on="Get status return code" class="DigNum (strict)"("Value"=w765) -> ()  [unwired: 2 in, 2 out]
                              n336 = Equal?(x=w766, y=w768) -> (x = y?=w767:bool)
                              n337 = property on="IDus not in read loop? (kinetic)" class="Bool (strict)"("Value"=FALSE ("IDus not in read loop? (kinetic)")) -> ()  [unwired: 2 in, 2 out]
                            }
                          }
                          frame #10 {
                            n338 = flat-sequence {
                              tunnel: [w775] -> w773
                              tunnel: w772 -> [w776]
                              tunnel: [w782] -> w774
                              tunnel: w771 -> [w779]
                              frame #0 {
                                n339 = Tick Count (ms)() -> (millisecond timer value=w777:u32)
                                n340 = Subtract(x=w777, y=w776) -> (x-y=w775:u32)
                                n341 = property on="Time  after the aquisition (before fetch data), (ms)" class="DigNum (strict)"("Value"=w775) -> ()  [unwired: 2 in, 2 out]
                              }
                              frame #1 {
                                n342 = call "GetAcquiredData.vi"("size"=w779) -> ("DLL error code"=w780:u32, "array"=w782:i32[])  [unwired: 2 in, 1 out]
                                n343 = Equal?(x=20002 ("DRV_SUCCESS"), y=w780) -> (x = y?=w778:bool)
                                n344 = property on="get aquired data return code" class="DigNum (strict)"("Value"=w780) -> ()  [unwired: 2 in, 2 out]
                                n345 = property on="Get aqisition ok? (kinetic mode)" class="Bool (strict)"("Value"=w778) -> ()  [unwired: 2 in, 2 out]
                              }
                            }
                            n346 = property on="Number of scans in kinetic cycle" class="DigNum (strict)"() -> ("Value"=w769:i32)  [unwired: 2 in, 2 out]
                            n347 = Multiply(x=1024.0, y=w769) -> (x*y=w771:dbl)
                          }
                          frame #11 {
                            n348 = Subtract(x=w793, y=w792) -> (x-y=w791:u32)
                            n349 = Divide(x=w791, y=w786) -> (x/y=w790:dbl)
                            n350 = for {
                              N: w786 -> [_]
                              tunnel: w794 -> [w808]
                              tunnel: w790 -> [w806]
                              tunnel: w789 -> [w804]
                              shift-right: [w802] -> w787
                              shift-left: w784 -> [w801]
                              shift-right: [w798] -> w788
                              shift-left: w785 -> [w799]
                              tunnel: w783 -> [_]
                              i -> [w796]
                              w803 = 1024 ("x")
                              n351 = Multiply(x=w796, y=w806) -> (x*y=w805:dbl)
                              n352 = Multiply(x=w803, y=w796) -> (x*y=w807:i32)
                              n353 = Add(x=w805, y=w804) -> (x+y=w800:dbl)
                              n354 = Array Subset(array=w808, index=w807, length=w803) -> (w795:i32[])
                              n355 = Equal To 0?(x=w796) -> (x = 0?=w797:bool)
                              n356 = case shown="True" w797 {
                                tunnel: w795 -> [_ w810]
                                frame False {
                                }
                                frame True {
                                n357 = for {
                                N: 1023 -> [_]
                                tunnel: [w813] -> w811 mode=indexing
                                i -> [w814]
                                n358 = Increment(x=w814) -> (x+1=w813:i32)
                                }
                                n359 = Bundle(w811, w810) -> (w809:cluster{i32[], i32[]})  [unwired: 1 in]
                                n360 = property class="XYGraph (strict)"("Value"=w809) -> ()  [unwired: 2 in, 2 out]
                                }
                              }
                              n361 = Build Array (concatenate)(w801, w795) -> (w802:dbl[][])
                              n362 = Build Array (concatenate)(w799, w800) -> (w798:dbl[])
                            }
                          }
                        }
                      }
                      frame "Wait" {
                        n363 = Unbundle By Name(w817) -> ("Sample rate"=w816:dbl)
                        n364 = Multiply(x=w816, y=1000.0) -> (x*y=w823:dbl)
                        n365 = Wait (ms)(milliseconds to wait=w823) -> ()  [unwired: 1 out]
                      }
                    }
                    n366 = case shown="True" w707 {
                      selector: w707 -> [_ w719]
                      frame False {
                      }
                      frame True {
                        n367 = property on="IDus not in read loop? (kinetic)" class="Bool (strict)"("Value"=w719) -> ()  [unwired: 2 in, 2 out]
                      }
                    }
                  }
                }
              }
              n368 = Bundle By Name(cluster=w569, "Time for spectrum measurment"=w583, "Time elapsed"=w584, "Spectrum"=w573) -> (w580:T11)
              n369 = Bundle By Name(cluster=w580, "Time for E measurment"=w582, "Potential array"=w581) -> (w575:T11)
            }
            frame "Read current and spectrum" {
              n370 = Unbundle By Name(w956) -> ("Time for spectrum measurment"=w970:i32[], "Start time"=w975:i32)
              n371 = Unbundle By Name(w956) -> ("Current array"=w969:dbl[])
              n372 = Unbundle By Name(w956) -> ("Time for I measurment"=w968:i32[], "Start time"=w974:i32)
              n373 = property on="V2 applied?" class="Bool (strict)"() -> ("Value"=w957:bool)  [unwired: 2 in, 2 out]
              n374 = case shown="False" w957 {
                tunnel: w956 -> [w991 w993]
                tunnel: [w990 w992] -> w955
                frame False {
                  n375 = Unbundle By Name(w991) -> ("V 1"=w990:dbl)
                }
                frame True {
                  n376 = Unbundle By Name(w993) -> ("V 2"=w992:dbl)
                }
              }
              n377 = local read "V (during measurment)"() -> (w976:dbl)
              n378 = Unbundle By Name(w956) -> ("V 1"=w977:dbl, "Spectrum"=w973:dbl[][])
              n379 = property on="Square wave?" class="Bool (strict)"() -> ("Value"=w962:bool)  [unwired: 2 in, 2 out]
              n380 = property on="V2 applied?" class="Bool (strict)"() -> ("Value"=w961:bool)  [unwired: 2 in, 2 out]
              n381 = property on="Use iDus?" class="Bool (strict)"() -> ("Value"=w967:bool)  [unwired: 2 in, 2 out]
              n382 = Equal?(x=w976, y=w977) -> (x = y?=w954:bool)
              n383 = And(x=w962, y=w961) -> (x .and. y?=w958:bool)
              n384 = Not(x=w958) -> (.not. x?=w960:bool)
              n385 = And(x=w954, y=w960) -> (x .and. y?=w959:bool)
              n386 = while {
                shift-right: [w1304] -> _
                shift-left: w956 -> [w1305]
                shift-right: [w1296] -> _
                shift-left: OSPEC-enum."Wait" -> [w1306]
                shift-right: [w1303] -> w980
                shift-left: w968 -> [w1302]
                shift-right: [w1297] -> w966
                shift-left: w969 -> [w1300]
                shift-right: [w1299] -> _
                shift-left: w974 -> [w1298]
                tunnel: w959 -> [w1295]
                shift-right: [w1293] -> w971
                shift-left: w972 -> [w1294]
                tunnel: w955 -> [w1289]
                i -> [w1301]
                stop <- w1290 stop-if-true
                n387 = case shown="\"Read\", Default" w1306 {
                  tunnel: w1305 -> [w1320 w1351 w1457]
                  tunnel: [w1319 w1351 w1457] -> w1304
                  tunnel: [w1317 FALSE FALSE] -> w1291
                  tunnel: [w1322 w1359 w1455] -> w1303
                  tunnel: w1302 -> [w1322 w1360 w1455]
                  tunnel: w1301 -> [_ w1365 _]
                  tunnel: [w1314 w1364 w1452] -> w1297
                  tunnel: w1300 -> [w1314 w1363 w1452]
                  tunnel: [w1312 w1352 w1454] -> w1299
                  tunnel: w1298 -> [w1312 _ w1454]
                  tunnel: [OSPEC-enum."Wait" OSPEC-enum."Check exit" OSPEC-enum."Read"] -> w1296
                  tunnel: w1295 -> [_ w1354 _]
                  tunnel: w1294 -> [w1313 w1346 w1451]
                  tunnel: [w1313 w1349 w1451] -> w1293
                  tunnel: w1289 -> [_ w1345 _]
                  frame "Check exit" {
                    n388 = local read "V (during measurment)"() -> (w1316:dbl)
                    n389 = property on="Square wave?" class="Bool (strict)"() -> ("Value"=w1310:bool)  [unwired: 2 in, 2 out]
                    n390 = property on="V2 applied?" class="Bool (strict)"() -> ("Value"=w1311:bool)  [unwired: 2 in, 2 out]
                    n391 = Unbundle By Name(w1320) -> ("V 1"=w1321:dbl)
                    n392 = Equal?(x=w1321, y=w1316) -> (x = y?=w1318:bool)
                    n393 = And(x=w1310, y=w1311) -> (x .and. y?=w1309:bool)
                    n394 = case shown="True" w1318 {
                      tunnel: w1320 -> [w1328 w1332]
                      tunnel: [w1328 w1332] -> w1319
                      tunnel: [w1327 w1331] -> w1317
                      tunnel: w1312 -> [w1326 w1330]
                      tunnel: w1309 -> [_ w1329]
                      frame False {
                        n395 = Unbundle By Name(w1328) -> ("V2 time"=w1324:dbl)
                        n396 = Multiply(x=1000.0, y=w1324) -> (x*y=w1325:dbl)
                        n397 = Greater Or Equal?(x=w1326, y=w1325) -> (x >= y?=w1327:bool)
                      }
                      frame True {
                        n398 = case shown="False" w1329 {
                          tunnel: w1332 -> [w1335 w1344]
                          tunnel: [w1333 w1343] -> w1331
                          tunnel: w1330 -> [w1334 w1342]
                          frame False {
                            n399 = Unbundle By Name(w1335) -> ("V1 time"=w1338:dbl)
                            n400 = Multiply(x=w1338, y=1000.0) -> (x*y=w1337:dbl)
                            n401 = Greater Or Equal?(x=w1334, y=w1337) -> (x >= y?=w1333:bool)
                          }
                          frame True {
                            n402 = Unbundle By Name(w1344) -> ("V off time"=w1340:dbl)
                            n403 = Multiply(x=w1340, y=1000.0) -> (x*y=w1341:dbl)
                            n404 = Greater Or Equal?(x=w1342, y=w1341) -> (x >= y?=w1343:bool)
                          }
                        }
                      }
                    }
                  }
                  frame "Read", Default {
                    # "Building a 1d matrix of currents"
                    n405 = property on="Use autolab?" class="Bool (strict)"() -> ("Value"=w1347:bool)  [unwired: 2 in, 2 out]
                    n406 = case shown="True" w1347 {
                      tunnel: [w1369 w1377] -> w1358
                      tunnel: [w1368 w1378] -> w1349
                      tunnel: w1346 -> [w1367 w1376]
                      tunnel: w1345 -> [_ w1379]
                      tunnel: w1345 -> [_ w1373]
                      tunnel: w1346 -> [_ w1375]
                      tunnel: w1345 -> [_ w1374]
                      frame False {
                        n407 = flat-sequence {
                          tunnel: w1367 -> [w1371]
                          tunnel: [w1370] -> w1366
                          frame #0 {
                            n408 = call "IV getcurrent.vi"("error in (no error)"=w1371) -> ("error out"=w1370:errorcluster, "value out"=w1372:dbl)  [unwired: 8 in, 1 out]
                            n409 = call "Current ranging routine (SubVI).vi"("Current"=w1372) -> ()  [unwired: 11 in]
                          }
                        }
                        n410 = call "IV getcurrent.vi"("error in (no error)"=w1366) -> ("error out"=w1368:errorcluster, "value out"=w1369:dbl)  [unwired: 8 in, 1 out]
                      }
                      frame True {
                        n411 = disable-structure shown="Enabled" {
                          disable-tunnel: w1379 -> [w1397 _]
                          disable-tunnel: [w1391 w1415] -> w1378
                          disable-tunnel: [w1389 w1414] -> w1377
                          disable-tunnel: w1376 -> [w1384 _]
                          disable-tunnel: w1375 -> [w1383 w1431]
                          disable-tunnel: w1374 -> [w1380 _]
                          disable-tunnel: w1373 -> [_ w1434]
                          frame Disabled {
                            n412 = property on="Ei" class="Ref (strict)"() -> ("Value"=w1381:refnum<k24>)  [unwired: 2 in, 2 out]
                            n413 = disable-structure shown="Disabled" {
                              disable-tunnel: w1397 -> [w1409 _]
                              disable-tunnel: [w1408 _] -> _
                              disable-tunnel: w1384 -> [w1405 _]
                              disable-tunnel: w1381 -> [w1404 _]
                              frame Disabled {
                                w1402 = 2 items=["UltraHigh_Speed", "High_Speed", "High_Stability"] ("Bandwidth")
                                w1407 = 1 items=["Off", "On"] ("CellOnOff")
                                w1403 = 0 items=["Potentiostatic", "Galvanostatic"] ("Mode")
                                n414 = property on="CurrentRange" class="DigNum (strict)"() -> ("Value"=w1406:i32)  [unwired: 2 in, 2 out]
                                n415 = property class="EI"(reference=w1404, error in=w1405, "Bandwidth"=w1402, "CellOnOff"=w1407, "CurrentRange"=w1406, "Mode"=w1403, "Setpoint"=w1409) -> (error out=w1408:errorcluster)  [unwired: 1 out]
                                n416 = property on="Sampler 2" class="Ref (strict)"(error in=w1408) -> (error out=w1401:errorcluster, "Value"=w1398:refnum<k24>)  [unwired: 1 in, 1 out]
                                n417 = property class="EI"(reference=w1404, error in=w1408) -> (error out=w1399:errorcluster, "EiStatusSupportedFor"=w1400:string[])  [unwired: 1 out]
                                n418 = invoke class="Sampler" method="Sample"(reference=w1398, error in=w1401) -> ()  [unwired: 1 in, 3 out]
                                n419 = property on="EI status supported for" class="Arr (strict)"(error in=w1399, "Value"=w1400) -> ()  [unwired: 1 in, 2 out]
                              }
                              frame Enabled {
                              }
                            }
                            n420 = property class="EI"(reference=w1381, error in=w1383, "Setpoint"=w1380) -> (error out=w1382:errorcluster)  [unwired: 1 out]
                            n421 = property class="EI" props=["Bandwidth", "CurrentRange", "Mode", "Setpoint", "Current", "Potential"](reference=w1381, error in=w1382) -> (error out=w1385:errorcluster, "Bandwidth"=w1396:i32, "CurrentRange"=w1395:i32, "Mode"=w1394:i32, "Current"=w1388:dbl, "Potential"=w1387:dbl)  [unwired: 2 out]
                            n422 = property on="Bandwidth" class="DigNum (strict)"("Value"=w1396) -> ()  [unwired: 2 in, 2 out]
                            n423 = property on="CurrentRange" class="DigNum (strict)"("Value"=w1395) -> ()  [unwired: 2 in, 2 out]
                            n424 = property on="Mode" class="DigNum (strict)"("Value"=w1394) -> ()  [unwired: 2 in, 2 out]
                            n425 = flat-sequence {
                              tunnel: [w1413] -> w1393
                              tunnel: w1388 -> [w1412]
                              tunnel: w1387 -> [w1411]
                              tunnel: [w1410] -> w1386
                              tunnel: w1385 -> [w1410]
                              frame #0 {
                                n426 = call "Range_selector.vi"("potential"=w1411, "current"=w1412) -> ("range integer"=w1413:i32)  [unwired: 9 in]
                              }
                            }
                            n427 = property class="EI"(reference=w1381, error in=w1386) -> (error out=w1392:errorcluster, "Current"=w1389:dbl, "Potential"=→"POtential PD":dbl)  [unwired: 1 out]
                            "Current PD" <- w1389
                            n428 = property class="EI"(reference=w1381, error in=w1392, "CurrentRange"=w1393) -> (error out=w1391:errorcluster)  [unwired: 1 out]
                          }
                          frame Enabled {
                            w1417 = 0 items=["Potentiostatic", "Galvanostatic"] ("Mode")
                            w1418 = 1 items=["Off", "On"] ("CellOnOff")
                            w1419 = 1 items=["UltraHigh_Speed", "High_Speed", "High_Stability"] ("Bandwidth")
                            w1424 = 1 items=["Off", "On"] ("CellOnOff")
                            w1425 = 1 items=["UltraHigh_Speed", "High_Speed", "High_Stability"] ("Bandwidth")
                            w1426 = 0 items=["Potentiostatic", "Galvanostatic"] ("Mode")
                            w1435 = 0 items=["Potentiostatic", "Galvanostatic"] ("Mode")
                            w1438 = 1 items=["Off", "On"] ("CellOnOff")
                            w1439 = 1 items=["UltraHigh_Speed", "High_Speed", "High_Stability"] ("Bandwidth")
                            n429 = property on="Sampler 2" class="Ref (strict)"() -> ("Value"=w1422:refnum<k24>)  [unwired: 2 in, 2 out]
                            n430 = property on="CurrentRange" class="DigNum (strict)"() -> ("Value"=w1437:i32)  [unwired: 2 in, 2 out]
                            n431 = property on="Ei" class="Ref (strict)"() -> ("Value"=w1421:refnum<k24>)  [unwired: 2 in, 2 out]
                            n432 = call "EI (A).vi"("Sampler"=w1422, "Ei"=w1421, "CellOnOff"=w1438, "Setpoint"=w1434, "Bandwidth"=w1439, "CurrentRange"=w1437, "Mode"=w1435, "error in (no error)"=w1431, "Disable Sampler"=FALSE) -> ("Cell"=w1432:bool, "Bandwidth"=w1433:i32, "error out"=w1430:errorcluster)  [unwired: 5 in, 11 out]
                            n433 = property on="Bandwidth" class="DigNum (strict)"("Value"=w1433) -> ()  [unwired: 2 in, 2 out]
                            n434 = property on="Cell on?" class="Bool (strict)"("Value"=w1432) -> ()  [unwired: 2 in, 2 out]
                            n435 = call "Sampler.vi"("error in (no error)"=w1431, "Sampler"=w1422) -> ("error out"=w1428:errorcluster)  [unwired: 7 in, 2 out]
                            n436 = Merge Errors(w1428, w1430) -> (w1429:errorcluster)
                            n437 = call "EI (A).vi"("Sampler"=w1422, "Ei"=w1421, "CellOnOff"=w1424, "Bandwidth"=w1425, "Mode"=w1426, "error in (no error)"=w1429, "Disable Sampler"=FALSE) -> ("Potential"=w1423:dbl, "Current"=w1414:dbl, "error out"=w1416:errorcluster)  [unwired: 7 in, 11 out]
                            "Current during PD" <- w1414
                            n438 = property on="Voltage" class="DigNum (strict)"("Value"=w1423) -> ()  [unwired: 2 in, 2 out]
                            n439 = property on="current" class="DigNum (strict)"("Value"=w1414) -> ()  [unwired: 2 in, 2 out]
                            n440 = call "Range_selector.vi"("potential"=w1423, "current"=w1414) -> ("range integer"=w1420:i32)  [unwired: 9 in]
                            n441 = call "EI (A).vi"("Sampler"=w1422, "Ei"=w1421, "CellOnOff"=w1418, "Bandwidth"=w1419, "CurrentRange"=w1420, "Mode"=w1417, "error in (no error)"=w1416) -> ("error out"=w1415:errorcluster)  [unwired: 7 in, 13 out]
                          }
                        }
                      }
                    }
                    n442 = Unbundle By Name(w1351) -> ("Start time"=w1350:i32)
                    n443 = Tick Count (ms)() -> (millisecond timer value=w1348:u32)
                    n444 = Subtract(x=w1348, y=w1350) -> (x-y=w1361:u32)
                    n445 = Equal?(x=1, y=w1365) -> (x = y?=w1355:bool)
                    n446 = And(x=w1354, y=w1355) -> (x .and. y?=w1353:bool)
                    n447 = case shown="True" w1353 {
                      tunnel: [w1441 w1445] -> w1359
                      tunnel: w1360 -> [w1442 w1443]
                      tunnel: w1361 -> [w1440 w1444]
                      tunnel: [w1440 w1444] -> w1352
                      frame False {
                        n448 = Build Array (concatenate)(w1442, w1440) -> (w1441:u32[])
                      }
                      frame True {
                        n449 = Build Array (concatenate)(w1443, w1444) -> (w1445:u32[])
                      }
                    }
                    n450 = case shown="True" w1353 {
                      tunnel: [w1447 w1449] -> w1364
                      tunnel: w1363 -> [w1448 _]
                      tunnel: w1358 -> [w1446 w1450]
                      frame False {
                        # "Intensity thereafter"
                        n451 = Build Array (concatenate)(w1448, w1446) -> (w1447:dbl[])
                      }
                      frame True {
                        n452 = Build Array(w1450) -> (w1449:dbl[])
                      }
                    }
                  }
                  frame "Wait" {
                    n453 = Unbundle By Name(w1457) -> ("Sample rate"=w1458:dbl)
                    n454 = Multiply(x=w1458, y=1000.0) -> (x*y=w1460:dbl)
                    n455 = Wait (ms)(milliseconds to wait=w1460) -> ()  [unwired: 1 out]
                  }
                }
                n456 = property on="Use iDus?" class="Bool (strict)"() -> ("Value"=w1288:bool)  [unwired: 2 in, 2 out]
                n457 = case shown="False" w1288 {
                  tunnel: [TRUE ("Value") w1308] -> w1292
                  frame False {
                  }
                  frame True {
                    n458 = property on="IDus not in read loop? (kinetic)" class="Bool (strict)"() -> ("Value"=w1308:bool)  [unwired: 2 in, 2 out]
                  }
                }
                n459 = And(x=w1292, y=w1291) -> (x .and. y?=w1290:bool)
              }
              n460 = case shown="False" w967 {
                tunnel: [w1007 w1115] -> w983
                tunnel: [w1006 w1117] -> w982
                tunnel: [w1001 w1114] -> w981
                tunnel: w975 -> [w1005 w1116]
                tunnel: w959 -> [w1004 w1120]
                tunnel: w973 -> [w1003 w1121]
                tunnel: w970 -> [w1002 w1119]
                tunnel: w956 -> [w995 w1118]
                tunnel: w954 -> [w994 w1113]
                tunnel: w958 -> [_ w1112]
                frame False {
                  n461 = case shown="True" w994 {
                    tunnel: w995 -> [_ w1017]
                    tunnel: [w1009 w1014] -> w1000
                    tunnel: [w1010 w1012] -> w998
                    tunnel: [w1011 w1013] -> w996
                    frame False {
                      n462 = property on="Wrapper Out" class="DigNum (strict)"() -> ("Value"=w1011:u32)  [unwired: 2 in, 2 out]
                      n463 = property on="ContinuousStrobe Out" class="DigNum (strict)"() -> ("Value"=w1010:u32)  [unwired: 2 in, 2 out]
                      n464 = property on="WL Values" class="Arr (strict)"() -> ("Value"=w1009:dbl[])  [unwired: 2 in, 2 out]
                    }
                    frame True {
                      n465 = Unbundle By Name(w1017) -> ("Continous strobe delay"=w1015:i32, "Integration time"=w1016:i32)
                      n466 = call "OSPEC-Open-Ocean.vi"("Integration Time"=w1016, "delay"=w1015) -> ("WL Values"=w1014:dbl[], "Wrapper Out"=w1013:u32, "ContinuousStrobe Out"=w1012:u32)  [unwired: 7 in]
                      "ContinuousStrobe Out" <- w1012
                      "Wrapper Out" <- w1013
                      "WL Values" <- w1014
                    }
                  }
                  n467 = while {
                    shift-right: [w1042] -> _
                    shift-left: w995 -> [w1043]
                    shift-right: [w1034] -> _
                    shift-left: OSPEC-enum."Wait" -> [w1044]
                    shift-right: [w1040] -> w1001
                    shift-left: w1002 -> [w1039]
                    shift-right: [w1032] -> w1006
                    shift-left: w1003 -> [w1038]
                    shift-right: [w1037] -> w1007
                    shift-left: w1005 -> [w1036]
                    tunnel: w1004 -> [w1033]
                    tunnel: w1000 -> [w1031]
                    tunnel: [w1030] -> w999
                    tunnel: w996 -> [w1027]
                    tunnel: w998 -> [w1028]
                    tunnel: [w1029] -> w997
                    i -> [w1035]
                    stop <- w1041 stop-if-true
                    n468 = case shown="\"Read\", Default" w1044 {
                      tunnel: w1043 -> [w1053 w1074 w1108]
                      tunnel: [w1052 w1074 w1108] -> w1042
                      tunnel: [w1050 FALSE FALSE] -> w1041
                      tunnel: [w1054 w1088 w1106] -> w1040
                      tunnel: w1039 -> [w1054 w1087 w1106]
                      tunnel: w1035 -> [_ w1082 _]
                      tunnel: [w1047 w1076 w1103] -> w1032
                      tunnel: w1038 -> [w1047 w1086 w1103]
                      tunnel: [w1051 w1077 w1105] -> w1037
                      tunnel: w1036 -> [w1051 _ w1105]
                      tunnel: [OSPEC-enum."Wait" OSPEC-enum."Check exit" OSPEC-enum."Read"] -> w1034
                      tunnel: w1033 -> [w1048 w1081 _]
                      tunnel: w1031 -> [_ w1067 _]
                      tunnel: [w1046 w1071 w1102] -> w1030
                      tunnel: w1028 -> [w1046 w1071 w1102]
                      tunnel: w1027 -> [w1045 w1070 w1101]
                      tunnel: [w1045 w1070 w1101] -> w1029
                      frame "Check exit" {
                        n469 = case shown="False" w1048 {
                          tunnel: w1053 -> [w1060 w1066]
                          tunnel: [w1060 w1066] -> w1052
                          tunnel: w1051 -> [w1058 w1064]
                          tunnel: [w1059 w1065] -> w1050
                          frame False {
                            n470 = Unbundle By Name(w1060) -> ("V2 time"=w1057:dbl)
                            n471 = Multiply(x=w1057, y=1000.0) -> (x*y=w1055:dbl)
                            n472 = Greater Or Equal?(x=w1058, y=w1055) -> (x >= y?=w1059:bool)
                          }
                          frame True {
                            n473 = Unbundle By Name(w1066) -> ("V1 time"=w1063:dbl)
                            n474 = Multiply(x=w1063, y=1000.0) -> (x*y=w1061:dbl)
                            n475 = Greater Or Equal?(x=w1064, y=w1061) -> (x >= y?=w1065:bool)
                          }
                        }
                      }
                      frame "Read", Default {
                        # "Check here to see if DIM t + 1 and DIM WL match"
                        n476 = Tick Count (ms)() -> (millisecond timer value=w1072:u32)
                        n477 = call "Wrapper_getSpectrum.vi"("Index"=0, "Wrapper"=w1070) -> ("Spectrum Values"=w1068:dbl[])  [unwired: 1 out]
                        n478 = Unbundle By Name(w1074) -> ("Start time"=w1073:i32)
                        n479 = Subtract(x=w1072, y=w1073) -> (x-y=w1078:u32)
                        n480 = Bundle("WL Values"=w1067, "Spectrum Values"=w1068) -> (→"?":T5)  [unwired: 1 in]
                        n481 = Equal?(x=w1082, y=1.0) -> (x = y?=w1080:bool)
                        n482 = And(x=w1081, y=w1080) -> (x .and. y?=w1079:bool)
                        n483 = case shown="False" w1079 {
                          tunnel: [w1091 w1092] -> w1076
                          tunnel: w1086 -> [w1090 _]
                          tunnel: w1068 -> [w1089 w1094]
                          tunnel: w1067 -> [_ w1093]
                          frame False {
                            # "Intensity thereafter"
                            n484 = Build Array (concatenate)(w1090, w1089) -> (w1091:dbl[][])
                          }
                          frame True {
                            n485 = Build Array(w1093, w1094) -> (w1092:dbl[][])
                          }
                        }
                        n486 = case shown="True" w1079 {
                          tunnel: [w1097 w1100] -> w1088
                          tunnel: w1087 -> [w1096 w1099]
                          tunnel: w1078 -> [w1095 w1098]
                          tunnel: [w1095 w1098] -> w1077
                          frame False {
                            n487 = Build Array (concatenate)(w1096, w1095) -> (w1097:u32[])
                          }
                          frame True {
                            n488 = Build Array (concatenate)(w1099, w1098) -> (w1100:u32[])
                          }
                        }
                      }
                      frame "Wait" {
                        n489 = Unbundle By Name(w1108) -> ("Sample rate"=w1109:dbl)
                        n490 = Multiply(x=w1109, y=1000.0) -> (x*y=w1111:dbl)
                        n491 = Wait (ms)(milliseconds to wait=w1111) -> ()  [unwired: 1 out]
                      }
                    }
                  }
                  n492 = disable-structure shown="Disabled" {
                    disable-tunnel: w999 -> [w1019 _]
                    disable-tunnel: w997 -> [w1018 _]
                    frame Disabled {
                      n493 = flat-sequence {
                        tunnel: [w1024] -> w1021
                        tunnel: [w1023] -> w1020
                        tunnel: w1019 -> [w1023]
                        tunnel: w1018 -> [w1022]
                        tunnel: w1021 -> [w1026]
                        tunnel: w1020 -> [w1025]
                        frame #0 {
                          # "Close spectrometers"
                          n494 = call "Wrapper_closeAllSpectrometers.vi"("Wrapper In"=w1022) -> ("Wrapper Out"=w1024:u32)
                        }
                        frame #1 {
                          # "Destroy \nwrapper \nand strobe"
                          n495 = call "ContinuousStrobe_Destroy.vi"("ContinuousStrobe"=w1025) -> ()
                          n496 = call "Wrapper_Destroy.vi"("Wrapper"=w1026) -> ()
                        }
                      }
                    }
                    frame Enabled {
                    }
                  }
                }
                frame True {
                  n497 = while {
                    shift-right: [w1135] -> w1115
                    shift-left: w1116 -> [w1136]
                    shift-right: [w1128] -> _
                    shift-left: OSPEC-enum."Wait" -> [w1137]
                    shift-right: [w1134] -> w1114
                    shift-left: w1119 -> [w1133]
                    shift-right: [w1126] -> w1117
                    shift-left: w1121 -> [w1132]
                    shift-right: [w1131] -> _
                    shift-left: w1118 -> [w1130]
                    tunnel: w1120 -> [w1127]
                    tunnel: w1113 -> [w1124]
                    tunnel: w1112 -> [w1123]
                    i -> [w1129]
                    stop <- w1125 stop-if-true
                    n498 = case shown="\"Read\", Default" w1137 {
                      tunnel: w1136 -> [w1146 _ w1285]
                      tunnel: [w1145 w1173 w1285] -> w1135
                      tunnel: [w1143 FALSE FALSE] -> w1125
                      tunnel: [w1147 w1174 w1283] -> w1134
                      tunnel: w1133 -> [w1147 w1179 w1283]
                      tunnel: w1129 -> [_ w1183 _]
                      tunnel: w1132 -> [w1141 w1177 w1279]
                      tunnel: [w1144 w1172 w1281] -> w1131
                      tunnel: w1130 -> [w1144 w1172 w1281]
                      tunnel: [OSPEC-enum."Wait" OSPEC-enum."Check exit" OSPEC-enum."Read"] -> w1128
                      tunnel: w1127 -> [_ w1178 _]
                      tunnel: [w1141 w1175 w1279] -> w1126
                      tunnel: w1124 -> [w1140 _ _]
                      tunnel: w1123 -> [w1139 _ _]
                      frame "Check exit" {
                        n499 = case shown="True" w1140 {
                          tunnel: w1146 -> [w1149 w1158]
                          tunnel: [w1149 w1157] -> w1145
                          tunnel: w1144 -> [w1148 w1156]
                          tunnel: [w1150 w1155] -> w1143
                          tunnel: w1139 -> [_ w1154]
                          frame False {
                            n500 = Unbundle By Name(w1148) -> ("V2 time"=w1151:dbl)
                            n501 = Multiply(x=w1151, y=1000.0) -> (x*y=w1152:dbl)
                            n502 = Greater Or Equal?(x=w1149, y=w1152) -> (x >= y?=w1150:bool)
                          }
                          frame True {
                            n503 = case shown="False" w1154 {
                              tunnel: w1158 -> [w1160 w1165]
                              tunnel: [w1160 w1165] -> w1157
                              tunnel: w1156 -> [w1159 w1166]
                              tunnel: [w1164 w1170] -> w1155
                              frame False {
                                n504 = Unbundle By Name(w1159) -> ("V1 time"=w1161:dbl)
                                n505 = Multiply(x=w1161, y=1000.0) -> (x*y=w1162:dbl)
                                n506 = Greater Or Equal?(x=w1160, y=w1162) -> (x >= y?=w1164:bool)
                              }
                              frame True {
                                n507 = Unbundle By Name(w1166) -> ("V off time"=w1167:dbl)
                                n508 = Multiply(x=w1167, y=1000.0) -> (x*y=w1168:dbl)
                                n509 = Greater Or Equal?(x=w1165, y=w1168) -> (x >= y?=w1170:bool)
                              }
                            }
                          }
                        }
                      }
                      frame "Read", Default {
                        n510 = Unbundle By Name(w1172) -> ("Start time"=w1171:i32)
                        n511 = property on="Number of scans in kinetic cycle" class="DigNum (strict)"() -> ("Value"=w1182:i32)  [unwired: 2 in, 2 out]
                        n512 = Tick Count (ms)() -> (millisecond timer value=w1180:u32)
                        n513 = Subtract(x=w1180, y=w1171) -> (x-y=w1173:u32)
                        n514 = call "GetDetector.vi"() -> ("xpixels"=w1181:i32)  [unwired: 4 in, 3 out]
                        n515 = Equal?(x=w1183, y=1.0) -> (x = y?=w1176:bool)
                        n516 = stacked-sequence {
                          seq-local: [_ _ _ _ _ _ _ _ _ _ w1217 _] -> [_ _ _ _ _ _ _ _ _ _ _ w1238]
                          seq-local: [_ _ _ _ _ _ _ _ w1202 _ _ _] -> [_ _ _ _ _ _ _ _ _ _ _ w1236]
                          seq-local: [_ _ _ _ _ _ _ _ _ _ w1216 _] -> [_ _ _ _ _ _ _ _ _ _ _ w1237]
                          tunnel: [_ _ _ _ _ _ _ _ _ _ _ w1231] -> w1175
                          tunnel: [_ _ _ _ _ _ _ _ _ _ _ w1232] -> w1174
                          tunnel: w1182 -> [_ _ _ _ _ w1195 _ _ _ _ w1213 w1230]
                          tunnel: w1173 -> [_ _ _ _ _ _ _ _ _ _ _ w1233]
                          tunnel: w1181 -> [_ w1188 _ _ _ _ _ _ _ _ _ _]
                          tunnel: w1171 -> [_ _ _ _ _ _ _ _ w1201 _ w1215 _]
                          tunnel: w1179 -> [_ _ _ _ _ _ _ _ _ _ _ w1229]
                          tunnel: w1178 -> [_ _ _ _ _ _ _ _ _ _ _ w1228]
                          tunnel: w1177 -> [_ _ _ _ _ _ _ _ _ _ _ w1227]
                          tunnel: w1176 -> [_ _ _ _ _ _ _ _ _ _ _ w1226]
                          frame #0 {
                            w1187 = u16 3  # AcquisitionMode
                            n517 = call "SetAcquisitionMode.vi"("mode"=w1187) -> ()  [unwired: 1 in, 2 out]
                          }
                          frame #1 {
                            w1189 = u16 0  # ReadMode
                            n518 = property on="xpixels" class="DigNum (strict)"("Value"=w1188) -> ()  [unwired: 2 in, 2 out]
                            n519 = call "SetReadMode.vi"("mode"=w1189) -> ()  [unwired: 1 in, 2 out]
                          }
                          frame #2 {
                            n520 = call "SetTriggerMode.vi"("mode"=TriggerMode_mode_typedef."Internal") -> ()  [unwired: 1 in, 2 out]
                          }
                          frame #3 {
                            n521 = property on="Exposure time (s)" class="DigNum (strict)"() -> ("Value"=w1191:dbl)  [unwired: 2 in, 2 out]
                            n522 = call "SetExposureTime.vi"("time"=w1191) -> ()  [unwired: 1 in, 2 out]
                          }
                          frame #4 {
                            n523 = call "GetNumberVSSpeeds.vi"() -> ("number"=w1194:i32)  [unwired: 3 in, 2 out]
                            n524 = Subtract(x=w1194, y=1) -> (x-y=w1192:i32)
                            n525 = call "SetVSSpeed.vi"("index"=w1192) -> ()  [unwired: 1 in, 2 out]
                          }
                          frame #5 {
                            n526 = call "SetNumberKinetics.vi"("number"=w1195) -> ()  [unwired: 1 in, 2 out]
                          }
                          frame #6 {
                            w1198 = 0  # Auto Shutter
                            n527 = call "SetShutter.vi"("type"="Shutter opens on TTL", "mode"=w1198, "closingtime"="Shutter open and close time", "openingtime"="Shutter open and close time") -> ()  [unwired: 10 in, 2 out]
                          }
                          frame #7 {
                            # "Meybe delete the exposure time insupt here"
                            n528 = property on="Exposure time (s)" class="DigNum (strict)"() -> ("Value"=w1199:dbl)  [unwired: 2 in, 2 out]
                            n529 = call "GetAcquisitionTimings.vi"("exposure input"=w1199) -> ("exposure"=w1200:sgl)  [unwired: 10 in, 4 out]
                            n530 = property on="Calculated exposure time" class="DigNum (strict)"("Value"=w1200) -> ()  [unwired: 2 in, 2 out]
                          }
                          frame #8 {
                            n531 = flat-sequence {
                              tunnel: [w1204] -> w1202
                              tunnel: w1201 -> [w1203]
                              frame #0 {
                                n532 = Tick Count (ms)() -> (millisecond timer value=w1205:u32)
                                n533 = Subtract(x=w1205, y=w1203) -> (x-y=w1204:u32)
                                "Time before the start of current aquisition (ms)" <- w1204
                              }
                              frame #1 {
                                n534 = call "StartAcquisition.vi"() -> ("DLL error code"=w1206:u32)  [unwired: 2 in, 1 out]
                                n535 = property on="Start Aquisition return code" class="DigNum (strict)"("Value"=w1206) -> ()  [unwired: 2 in, 2 out]
                              }
                            }
                          }
                          frame #9 {
                            n536 = while {
                              stop <- w1210 continue-if-true
                              w1211 = u16 72  # DRV ACQUIRING
                              n537 = call "GetStatus.vi"() -> ("DLL error code"=w1208:u32, "status"=w1209:T18)  [unwired: 3 in, 1 out]
                              n538 = property on="Get status return code" class="DigNum (strict)"("Value"=w1208) -> ()  [unwired: 2 in, 2 out]
                              n539 = Equal?(x=w1209, y=w1211) -> (x = y?=w1210:bool)
                              "IDus not in read loop? (kinetic)" <- FALSE
                            }
                          }
                          frame #10 {
                            n540 = flat-sequence {
                              tunnel: [w1218] -> w1216
                              tunnel: w1215 -> [w1219]
                              tunnel: [w1225] -> w1217
                              tunnel: w1214 -> [w1221]
                              frame #0 {
                                n541 = Tick Count (ms)() -> (millisecond timer value=w1220:u32)
                                n542 = Subtract(x=w1220, y=w1219) -> (x-y=w1218:u32)
                                "Time  after the aquisition (before fetch data), (ms)" <- w1218
                              }
                              frame #1 {
                                n543 = call "GetAcquiredData.vi"("size"=w1221) -> ("DLL error code"=w1222:u32, "array"=w1225:i32[])  [unwired: 2 in, 1 out]
                                n544 = Equal?(x=20002 ("DRV_SUCCESS"), y=w1222) -> (x = y?=→"Get aqisition ok? (kinetic mode)":bool)
                                n545 = property on="get aquired data return code" class="DigNum (strict)"("Value"=w1222) -> ()  [unwired: 2 in, 2 out]
                              }
                            }
                            n546 = Multiply(x=1024, y=w1213) -> (x*y=w1214:i32)
                          }
                          frame #11 {
                            n547 = Subtract(x=w1237, y=w1236) -> (x-y=w1235:u32)
                            n548 = Divide(x=w1235, y=w1230) -> (x/y=w1234:dbl)
                            n549 = for {
                              N: w1230 -> [_]
                              tunnel: w1238 -> [w1256]
                              tunnel: w1234 -> [w1254]
                              tunnel: w1233 -> [w1251]
                              shift-right: [w1249] -> w1231
                              shift-left: w1227 -> [w1248]
                              shift-right: [w1241] -> w1232
                              shift-left: w1229 -> [w1246]
                              tunnel: w1228 -> [w1244]
                              tunnel: w1226 -> [w1242]
                              i -> [w1240]
                              w1250 = 1024 ("x")
                              n550 = Equal To 0?(x=w1240) -> (x = 0?=w1239:bool)
                              n551 = Multiply(x=w1240, y=w1254) -> (x*y=w1253:dbl)
                              n552 = Multiply(x=w1250, y=w1240) -> (x*y=w1255:i32)
                              n553 = Add(x=w1253, y=w1251) -> (x+y=w1247:dbl)
                              n554 = Array Subset(array=w1256, index=w1255, length=w1250) -> (w1252:i32[])
                              n555 = And(x=w1239, y=w1242) -> (x .and. y?=w1243:bool)
                              n556 = And(x=w1244, y=w1243) -> (x .and. y?=w1245:bool)
                              n557 = case shown="False" w1245 {
                                tunnel: w1252 -> [w1257 w1270]
                                tunnel: [w1262 w1273] -> w1249
                                tunnel: w1248 -> [w1263 _]
                                tunnel: w1247 -> [w1260 w1275]
                                tunnel: [w1259 w1274] -> w1241
                                tunnel: w1246 -> [w1261 _]
                                tunnel: w1239 -> [w1258 _]
                                frame False {
                                n558 = case shown="True" w1258 {
                                tunnel: w1257 -> [_ w1266]
                                frame False {
                                }
                                frame True {
                                n559 = for {
                                N: 1023 -> [_]
                                tunnel: [w1268] -> _ mode=indexing
                                tunnel: [w1268] -> w1265 mode=indexing
                                i -> [w1269]
                                n560 = Increment(x=w1269) -> (x+1=w1268:i32)
                                }
                                n561 = Bundle(w1265, w1266) -> (w1264:cluster{i32[], i32[]})  [unwired: 1 in]
                                n562 = property class="XYGraph (strict)"("Value"=w1264) -> ()  [unwired: 2 in, 2 out]
                                }
                                }
                                n563 = Build Array (concatenate)(w1263, w1257) -> (w1262:dbl[][])
                                n564 = Build Array (concatenate)(w1261, w1260) -> (w1259:dbl[])
                                }
                                frame True {
                                n565 = for {
                                N: 1023 -> [_]
                                tunnel: [w1277] -> w1271 mode=indexing
                                i -> [w1278]
                                n566 = Increment(x=w1278) -> (x+1=w1277:i32)
                                }
                                n567 = Bundle(w1271, w1270) -> (w1272:cluster{i32[], i32[]})  [unwired: 1 in]
                                n568 = Build Array(w1275) -> (w1274:dbl[])
                                n569 = Build Array(w1271, w1270) -> (w1273:i32[][])
                                n570 = property class="XYGraph (strict)"("Value"=w1272) -> ()  [unwired: 2 in, 2 out]
                                }
                              }
                            }
                          }
                        }
                      }
                      frame "Wait" {
                        n571 = Unbundle By Name(w1281) -> ("Sample rate"=w1280:dbl)
                        n572 = Multiply(x=w1280, y=1000.0) -> (x*y=w1287:dbl)
                        n573 = Wait (ms)(milliseconds to wait=w1287) -> ()  [unwired: 1 out]
                      }
                    }
                    n574 = case shown="True" w1125 {
                      frame False {
                      }
                      frame True {
                        n575 = property on="IDus not in read loop? (kinetic)" class="Bool (strict)"("Value"=TRUE ("IDus not in read loop? (kinetic)")) -> ()  [unwired: 2 in, 2 out]
                      }
                    }
                  }
                }
              }
              n576 = Bundle By Name(cluster=w956, "Time for spectrum measurment"=w981, "Time elapsed"=w983, "Spectrum"=w982) -> (w978:T11)
              n577 = Bundle By Name(cluster=w978, "Time for I measurment"=w980, "Current array"=w966) -> (w979:T11)
              n578 = local read "V (during measurment)"() -> (w985:dbl)
              n579 = property on="V2 applied?" class="Bool (strict)"() -> ("Value"=w965:bool)  [unwired: 2 in, 2 out]
              n580 = Unbundle By Name(w978) -> ("V 1"=w986:dbl)
              n581 = Equal?(x=w986, y=w985) -> (x = y?=w987:bool)
              n582 = And(x=w965, y="Square wave?") -> (x .and. y?=w964:bool)
              n583 = case shown="False" w987 {
                tunnel: [w1462 w1466] -> w988
                tunnel: w964 -> [_ w1465]
                tunnel: "Square wave?" -> [w1461 _]
                frame False {
                  n584 = case shown="False" w1461 {
                    tunnel: [OSSPEC."Read Potential and spectrum" OSSPEC."Apply V1"] -> w1462
                    frame False {
                    }
                    frame True {
                    }
                  }
                }
                frame True {
                  n585 = case shown="False" w1465 {
                    tunnel: [OSSPEC."Apply V2" OSSPEC."End measurment"] -> w1466
                    frame False {
                    }
                    frame True {
                    }
                  }
                }
              }
            }
            frame "Reinitialise Cell" {
              # "this state is no longer used as it adds a 1-300 ms delay before the spectrum is measured as the mode is shifted"
              n586 = flat-sequence {
                tunnel: w1475 -> [w1479]
                tunnel: [w1478] -> w1470
                tunnel: w1470 -> [w1482]
                tunnel: [w1481] -> w1469
                tunnel: [w1483] -> w1474
                tunnel: w1469 -> [w1483]
                frame #0 {
                  n587 = To Long Integer(number=T17."IStat4EL" ("Configuration")) -> (32bit integer=w1477:i32)
                  n588 = call "IV setconnectionmode.vi"("error in (no error)"=w1479, "value"=w1477) -> ("error out"=w1478:errorcluster)  [unwired: 7 in, 2 out]
                }
                frame #1 {
                  n589 = call "IV setcurrent.vi"("error in (no error)"=w1482, "value"=0.0) -> ("error out"=w1481:errorcluster)  [unwired: 7 in, 2 out]
                }
                frame #2 {
                }
              }
              n590 = Unbundle By Name(w1471) -> ()  [unwired: 3 out]
            }
            frame "Apply V1" {
              n591 = property on="Use autolab?" class="Bool (strict)"() -> ("Value"=w1487:bool)  [unwired: 2 in, 2 out]
              n592 = property on="Potential  During PD" class="WFChart (strict)"("History Data"=dbl[] []) -> ()  [unwired: 2 in, 2 out]
              n593 = property on="Current during PD" class="WFChart (strict)"("History Data"=dbl[] []) -> ()  [unwired: 2 in, 2 out]
              n594 = flat-sequence {
                tunnel: w1495 -> [w1501]
                tunnel: w1494 -> [w1500]
                tunnel: [w1499] -> w1489
                tunnel: [w1498] -> w1488
                tunnel: w1487 -> [w1497]
                tunnel: [w1496] -> w1486
                tunnel: w1495 -> [w1542]
                tunnel: w1489 -> [w1540]
                tunnel: [w1541] -> w1491
                tunnel: [w1536] -> w1490
                tunnel: w1488 -> [w1535]
                tunnel: w1487 -> [w1534]
                tunnel: w1486 -> [w1533]
                frame #0 {
                  n595 = case shown="True" w1497 {
                    tunnel: w1501 -> [w1507 w1524]
                    tunnel: w1500 -> [w1506 _]
                    tunnel: [w1505 w1516] -> w1499
                    tunnel: [w1503 w1523] -> w1498
                    tunnel: [refnum<k24> refnum ("Value") w1520] -> w1496
                    frame False {
                      n596 = Unbundle By Name(w1507) -> ("V 1"=w1505:dbl)
                      n597 = Absolute Value(x=w1505) -> (abs(x)=w1509:dbl)
                      n598 = local write "V (during measurment)"(w1505) -> ()
                      n599 = Greater?(x=w1509, y=3.0) -> (0:w1508:bool)
                      n600 = case shown="False" w1508 {
                        tunnel: [w1510 w1512] -> w1503
                        tunnel: w1506 -> [w1510 w1511]
                        frame False {
                        }
                        frame True {
                          # "abort if E >3 V"
                          n601 = call "IV setcellon.vi"("error in (no error)"=w1511, "cellon"=0) -> ("error out"=w1514:errorcluster)  [unwired: 7 in, 2 out]
                          n602 = call "IV close.vi"("error in (no error)"=w1514) -> ("error out"=w1512:errorcluster)  [unwired: 9 in, 1 out]
                          n603 = call "Display Message to User3"("error in (no error)"=w1512) -> ("OK"=w1515:bool)  [unwired: 9 in, 1 out]
                          n604 = Stop(stop? (T)=w1515) -> ()
                        }
                      }
                    }
                    frame True {
                      w1530 = 1 items=["Off", "On"] ("CellOnOff")
                      n605 = property on="Ei" class="Ref (strict)"() -> ("Value"=w1520:refnum<k24>)  [unwired: 2 in, 2 out]
                      n606 = property on="Sampler 2" class="Ref (strict)"() -> ("Value"=w1526:refnum<k24>)  [unwired: 2 in, 2 out]
                      n607 = property class="EI" props=["EiStatusSupportedFor"](reference=w1520) -> (error out=w1522:errorcluster)  [unwired: 1 in, 2 out]
                      n608 = property class="EI" props=["Bandwidth", "CurrentRange", "Mode", "Potential", "Current"](reference=w1520) -> (error out=w1528:errorcluster, "Potential"=w1532:dbl, "Current"=w1531:dbl)  [unwired: 1 in, 4 out]
                      n609 = invoke class="Sampler" method="Sample"(reference=w1526) -> (error out=w1521:errorcluster)  [unwired: 2 in, 2 out]
                      n610 = Unbundle By Name(w1524) -> ("V 1"=w1516:dbl)
                      n611 = call "Range_selector.vi"("potential"=w1532, "current"=w1531) -> ("range integer"=w1529:i32)  [unwired: 9 in]
                      n612 = property class="EI"(reference=w1520, error in=w1528, "CellOnOff"=w1530, "CurrentRange"=w1529) -> (error out=w1527:errorcluster)  [unwired: 1 out]
                      n613 = call "P_Stat_Status1.vi"("error in (no error)"=w1527, ".NET Refnum in"=w1520) -> ("error out"=w1525:errorcluster, "PotentialOverload"=w1517:bool, "CurrentOverload"=w1519:bool, "Cell"=w1518:bool)  [unwired: 3 in, 3 out]
                      n614 = Merge Errors(w1525, w1522, w1521) -> (w1523:errorcluster)
                      n615 = property on="V (during measurment)" class="DigNum (strict)"("Value"=w1516) -> ()  [unwired: 2 in, 2 out]
                      n616 = property on="Cell on?" class="Bool (strict)"("Value"=w1518) -> ()  [unwired: 2 in, 2 out]
                      n617 = property on="PotentialOverload" class="Bool (strict)"("Value"=w1517) -> ()  [unwired: 2 in, 2 out]
                      n618 = property on="CurrentOverload" class="Bool (strict)"("Value"=w1519) -> ()  [unwired: 2 in, 2 out]
                    }
                  }
                }
                frame #1 {
                  n619 = property on="Square wave?" class="Bool (strict)"() -> ("Value"=w1538:bool)  [unwired: 2 in, 2 out]
                  n620 = property on="V2 applied?" class="Bool (strict)"() -> ("Value"=w1539:bool)  [unwired: 2 in, 2 out]
                  n621 = case shown="True" w1534 {
                    tunnel: w1540 -> [w1545 w1548]
                    tunnel: [w1544 w1547] -> w1536
                    tunnel: w1535 -> [w1543 w1549]
                    tunnel: w1533 -> [_ w1546]
                    frame False {
                      n622 = call "IV setpotential.vi"("error in (no error)"=w1543, "value"=w1545) -> ("error out"=w1544:errorcluster)  [unwired: 7 in, 2 out]
                    }
                    frame True {
                      n623 = property class="EI"(reference=w1546, error in=w1549, "Setpoint"=w1548) -> (error out=w1547:errorcluster)  [unwired: 1 out]
                    }
                  }
                  n624 = And(x=w1538, y=w1539) -> (x .and. y?=w1537:bool)
                  n625 = case shown="False" w1537 {
                    tunnel: w1542 -> [w1553 w1554]
                    tunnel: [w1552 w1554] -> w1541
                    frame False {
                      n626 = Tick Count (ms)() -> (millisecond timer value=w1550:u32)
                      n627 = Bundle By Name(cluster=w1553, "Start time"=w1550, "Time elapsed"=0) -> (w1552:T11)
                    }
                    frame True {
                    }
                  }
                }
              }
            }
            frame "Apply V2" {
              n628 = Tick Count (ms)() -> (millisecond timer value=w1562:u32)
              n629 = flat-sequence {
                tunnel: w1557 -> [w1575]
                tunnel: [w1576] -> w1568
                tunnel: w1567 -> [w1574]
                tunnel: [w1569] -> w1564
                tunnel: [w1573] -> w1563
                tunnel: w1562 -> [w1573]
                tunnel: w1557 -> [w1572]
                tunnel: [w1571] -> w1556
                tunnel: [w1570] -> w1555
                tunnel: w1568 -> [w1612]
                tunnel: w1564 -> [w1611]
                tunnel: w1563 -> [w1610]
                tunnel: [w1610] -> w1560
                tunnel: [w1609] -> w1558
                tunnel: w1556 -> [w1607]
                tunnel: w1555 -> [w1606]
                frame #0 {
                  n630 = property on="Use autolab?" class="Bool (strict)"() -> ("Value"=w1571:bool)  [unwired: 2 in, 2 out]
                  n631 = Unbundle By Name(w1575) -> ("V 2"=w1569:dbl)
                  n632 = Absolute Value(x=w1569) -> (abs(x)=w1579:dbl)
                  n633 = Greater?(x=w1579, y=3.0) -> (0:w1577:bool)
                  n634 = local write "V (during measurment)"(w1569) -> ()
                  n635 = case shown="False" w1571 {
                    tunnel: w1577 -> [w1583 _]
                    tunnel: [w1582 w1596] -> w1576
                    tunnel: w1574 -> [w1581 _]
                    tunnel: w1572 -> [_ _]
                    tunnel: [refnum<k24> refnum ("Value") w1595] -> w1570
                    tunnel: w1569 -> [_ w1593]
                    frame False {
                      n636 = case shown="True" w1583 {
                        tunnel: [w1584 w1586] -> w1582
                        tunnel: w1581 -> [w1584 w1585]
                        frame False {
                        }
                        frame True {
                          # "abort if E >3 V"
                          n637 = call "IV setcellon.vi"("error in (no error)"=w1585, "cellon"=0) -> ("error out"=w1588:errorcluster)  [unwired: 7 in, 2 out]
                          n638 = call "IV close.vi"("error in (no error)"=w1588) -> ("error out"=w1586:errorcluster)  [unwired: 9 in, 1 out]
                          n639 = call "Display Message to User4"("error in (no error)"=w1586) -> ("OK"=w1589:bool)  [unwired: 9 in, 1 out]
                          n640 = Stop(stop? (T)=w1589) -> ()
                        }
                      }
                    }
                    frame True {
                      w1603 = 1 items=["Off", "On"] ("CellOnOff")
                      n641 = property on="Ei" class="Ref (strict)"() -> ("Value"=w1595:refnum<k24>)  [unwired: 2 in, 2 out]
                      n642 = property on="Sampler 2" class="Ref (strict)"() -> ("Value"=w1597:refnum<k24>)  [unwired: 2 in, 2 out]
                      n643 = property class="EI"(reference=w1595) -> (error out=w1594:errorcluster, "EiStatusSupportedFor"=w1592:string[])  [unwired: 1 in, 1 out]
                      n644 = property class="EI" props=["Bandwidth", "CurrentRange", "Mode", "Potential", "Current"](reference=w1595) -> (error out=w1601:errorcluster, "Potential"=w1605:dbl, "Current"=w1604:dbl)  [unwired: 1 in, 4 out]
                      n645 = invoke class="Sampler" method="Sample"(reference=w1597) -> (error out=w1598:errorcluster)  [unwired: 2 in, 2 out]
                      n646 = call "Range_selector.vi"("potential"=w1605, "current"=w1604) -> ("range integer"=w1602:i32)  [unwired: 9 in]
                      n647 = property class="EI"(reference=w1595, error in=w1601, "CellOnOff"=w1603, "CurrentRange"=w1602, "Setpoint"=w1593) -> (error out=w1600:errorcluster)  [unwired: 1 out]
                      n648 = property on="EI status supported for" class="Arr (strict)"("Value"=w1592) -> ()  [unwired: 2 in, 2 out]
                      n649 = call "P_Stat_Status1.vi"("error in (no error)"=w1600, ".NET Refnum in"=w1595) -> ("error out"=w1599:errorcluster, "PotentialOverload"=w1590:bool, "CurrentOverload"=w1591:bool)  [unwired: 3 in, 4 out]
                      n650 = property on="CurrentOverload" class="Bool (strict)"("Value"=w1591) -> ()  [unwired: 2 in, 2 out]
                      n651 = Merge Errors(w1599, w1594, w1598) -> (w1596:errorcluster)
                      n652 = property on="PotentialOverload" class="Bool (strict)"("Value"=w1590) -> ()  [unwired: 2 in, 2 out]
                    }
                  }
                }
                frame #1 {
                  n653 = case shown="False" w1607 {
                    tunnel: w1612 -> [w1615 w1618]
                    tunnel: w1611 -> [w1614 w1616]
                    tunnel: [w1613 w1617] -> w1609
                    tunnel: w1606 -> [_ w1619]
                    frame False {
                      n654 = call "IV setpotential.vi"("error in (no error)"=w1615, "value"=w1614) -> ("error out"=w1613:errorcluster)  [unwired: 7 in, 2 out]
                    }
                    frame True {
                      n655 = property class="EI"(reference=w1619, error in=w1618, "Setpoint"=w1616) -> (error out=w1617:errorcluster)  [unwired: 1 out]
                    }
                  }
                  "V2 applied?" <- TRUE ("V2 applied")
                }
              }
              n656 = Tick Count (ms)() -> (millisecond timer value=w1559:u32)
              n657 = Subtract(x=w1559, y=w1560) -> (x-y=→"Time taken to apply V2":u32)
              n658 = Unbundle By Name(w1557) -> ()  [unwired: 3 out]
            }
            frame "End measurment" {
              w1630 = ext 0.00099999999999999999996
              w1647 = TRUE
              n659 = Unbundle By Name(w1620) -> ("Time for spectrum measurment"=w1626:i32[], "Spectrum"=w1643:dbl[][])
              n660 = Unbundle By Name(w1620) -> ("Current array"=w1637:dbl[], "Time for I measurment"=w1632:i32[])
              n661 = Unbundle By Name(w1620) -> ("Time for E measurment"=w1629:i32[], "Potential array"=w1638:dbl[])
              n662 = Multiply(x=w1626, y=ext 0.00099999999999999999996) -> (x*y=w1625:ext[])
              n663 = Multiply(x=w1632, y=w1630) -> (x*y=w1631:ext[])
              n664 = Multiply(x=w1630, y=w1629) -> (x*y=w1628:ext[])
              n665 = Build Array(w1631, w1637) -> (w1636:ext[][])
              n666 = Build Array(w1628, w1638) -> (w1634:ext[][])
              n667 = Insert Into Array(array=w1625, index=0, new element=0 ("new element/subarray")) -> (w1641:ext[])
              n668 = Transpose 2D Array(2D array=w1636) -> (transposed array=w1635:ext[][])
              n669 = Transpose 2D Array(2D array=w1634) -> (transposed array=w1633:ext[][])
              n670 = Insert Into Array(array=w1643, index (col)=0 ("disabled index (col)"), new element=w1641) -> (w1640:dbl[][])  [unwired: 1 in]
              n671 = call "Write-OSP-J-t.vi"("Init cluster"=w1620, "Array"=w1635) -> ()  [unwired: 10 in]
              n672 = call "Write-OSP-E-t.vi"("Init cluster"=w1620, "Array"=w1633) -> ()  [unwired: 10 in]
              n673 = Transpose 2D Array(2D array=w1640) -> (transposed array=w1639:dbl[][])
              n674 = call "Write-OSP-SP.vi"("Init cluster"=w1620, "Array"=w1639) -> ()  [unwired: 10 in]
              n675 = property on="T reached?" class="Bool (strict)"("Value"=FALSE ("T reached?")) -> ()  [unwired: 2 in, 2 out]
              n676 = Unbundle By Name(w1620) -> ("Default\n potential"=w1622:dbl)
              n677 = property on="Use autolab?" class="Bool (strict)"() -> ("Value"=w1623:bool)  [unwired: 2 in, 2 out]
              n678 = case shown="True" w1623 {
                tunnel: w1622 -> [w1651 w1667]
                tunnel: w1648 -> [w1650 w1666]
                tunnel: [w1649 w1665] -> w1646
                frame False {
                  n679 = flat-sequence {
                    tunnel: w1650 -> [w1655]
                    tunnel: [w1654] -> w1653
                    tunnel: w1651 -> [w1660]
                    tunnel: w1653 -> [w1659]
                    tunnel: [w1658] -> w1652
                    tunnel: w1652 -> [w1662]
                    tunnel: [w1661] -> w1649
                    frame #0 {
                      n680 = To Long Integer(number=T17."EStat4EL" ("Configuration")) -> (32bit integer=w1657:i32)
                      n681 = call "IV setconnectionmode.vi"("error in (no error)"=w1655, "value"=w1657) -> ("error out"=w1654:errorcluster)  [unwired: 7 in, 2 out]
                    }
                    frame #1 {
                      n682 = call "IV setpotential.vi"("error in (no error)"=w1659, "value"=w1660) -> ("error out"=w1658:errorcluster)  [unwired: 7 in, 2 out]
                    }
                    frame #2 {
                      n683 = call "IV getcurrent.vi"("error in (no error)"=w1662) -> ("error out"=w1661:errorcluster, "value out"=w1663:dbl)  [unwired: 8 in, 1 out]
                      n684 = call "Current ranging routine (SubVI).vi"("Current"=w1663) -> ()  [unwired: 11 in]
                    }
                  }
                }
                frame True {
                  w1672 = 0 items=["Off", "On"] ("CellOnOff")
                  n685 = property on="Ei" class="Ref (strict)"() -> ("Value"=w1664:refnum<k24>)  [unwired: 2 in, 2 out]
                  n686 = disable-structure shown="Enabled" {
                    disable-tunnel: [w1692 _] -> w1670
                    disable-tunnel: [w1691 _] -> w1669
                    disable-tunnel: [w1690 -3 ("range integer")] -> w1668
                    disable-tunnel: w1667 -> [w1688 _]
                    disable-tunnel: w1666 -> [w1686 _]
                    disable-tunnel: w1664 -> [w1681 _]
                    frame Disabled {
                      w1687 = -2 items=["CR07_1A"=0, "CR06_10A"=1, "CR01_100A"=2, "CR00_1000A"=3, "CR05_20A"=20, "CR04_40A"=40, "CR03_50A"=60, "CR02_80A"=80, "CR19_1pA"=-12, "CR18_10pA"=-11, "CR17_100pA"=-10, "CR16_1nA"=-9, "CR15_10nA"=-8, "CR14_100nA"=-7, "CR13_1uA"=-6, "CR12_10uA"=-5, "CR11_100uA"=-4, "CR10_1mA"=-3, "CR09_10mA"=-2, "CR08_100mA"=-1] ("CurrentRange")
                      w1689 = 0 items=["Potentiostatic", "Galvanostatic"] ("Mode")
                      n687 = property class="EI"(reference=w1681, error in=w1686, "Setpoint"=w1688, "Mode"=w1689, "CurrentRange"=w1687) -> (error out=w1683:errorcluster)  [unwired: 1 out]
                      n688 = property on="Sampler 2" class="Ref (strict)"() -> ("Value"=w1682:refnum<k24>)  [unwired: 2 in, 2 out]
                      n689 = property class="EI"(reference=w1681, error in=w1683) -> ("Current"=w1684:dbl, "Potential"=w1685:dbl)  [unwired: 2 out]
                      n690 = property class="EI" props=["EiStatusSupportedFor"](reference=w1681) -> (error out=w1692:errorcluster)  [unwired: 1 in, 2 out]
                      n691 = invoke class="Sampler" method="Sample"(reference=w1682) -> (error out=w1691:errorcluster)  [unwired: 2 in, 2 out]
                      n692 = flat-sequence {
                        tunnel: [w1696] -> w1690
                        tunnel: w1685 -> [w1695]
                        tunnel: w1684 -> [w1694]
                        frame #0 {
                          n693 = Wait (ms)(milliseconds to wait=u32 50) -> ()  [unwired: 1 out]
                        }
                        frame #1 {
                          n694 = call "Range_selector.vi"("potential"=w1695, "current"=w1694) -> ("range integer"=w1696:i32)  [unwired: 9 in]
                        }
                      }
                    }
                    frame Enabled {
                    }
                  }
                  n695 = property class="EI"(reference=w1664, "CellOnOff"=w1672, "CurrentRange"=w1668) -> (error out=w1671:errorcluster)  [unwired: 1 in, 1 out]
                  n696 = disable-structure shown="Enabled" {
                    disable-tunnel: w1671 -> [w1680 _]
                    disable-tunnel: w1670 -> [w1678 _]
                    disable-tunnel: w1669 -> [w1677 _]
                    disable-tunnel: [w1676 _] -> w1665
                    disable-tunnel: w1664 -> [w1675 _]
                    frame Disabled {
                      n697 = call "P_Stat_Status1.vi"("error in (no error)"=w1680, ".NET Refnum in"=w1675) -> ("error out"=w1679:errorcluster, "PotentialOverload"=w1674:bool, "CurrentOverload"=w1673:bool)  [unwired: 3 in, 4 out]
                      n698 = property on="CurrentOverload" class="Bool (strict)"("Value"=w1673) -> ()  [unwired: 2 in, 2 out]
                      n699 = Merge Errors(w1679, w1678, w1677) -> (w1676:errorcluster)
                      n700 = property on="PotentialOverload" class="Bool (strict)"("Value"=w1674) -> ()  [unwired: 2 in, 2 out]
                    }
                    frame Enabled {
                    }
                  }
                }
              }
              "PD ENDED\nEXIT MEASURMENT" <- w1647
            }
          }
        }
        n701 = property on="PD ENDED\nEXIT MEASURMENT" class="Bool (strict)"() -> ("Value"=w535:bool)  [unwired: 2 in, 2 out]
        n702 = case shown="True" w535 {
          tunnel: [State."Wait for Event" ("f") State."Exit" ("f")] -> w544
          frame False {
          }
          frame True {
          }
        }
      }
      frame "Initialse and cool iDus" {
        # "Also re-intialise constants"
        n703 = Unbundle By Name(w1699) -> ("Return detector to \nroom T"=w1702:bool)
        n704 = case shown="False" w1702 {
          tunnel: [State."Wait for Event" ("f") State."Wait for Event" ("f")] -> w1701
          frame False {
            w1711 = 20002  # DRV_SUCCESS
            n705 = stacked-sequence {
              seq-local: [_ _ _ _ _ _ w1777] -> [_ _ _ _ _ _ _]
              seq-local: [_ _ _ _ _ _ w1778] -> [_ _ _ _ _ _ _]
              tunnel: w1711 -> [w1767 _ _ _ _ _ _]
              tunnel: [w1766 _ _ _ _ _ _] -> w1710
              tunnel: [_ _ _ _ _ _ w1777] -> _
              tunnel: [_ _ _ _ _ _ w1778] -> w1705
              frame #0 {
                n706 = call "Initialize.vi"("directory (\"\")"="" ("directory (\"\")")) -> ("DLL error code"=w1769:u32)  [unwired: 1 in, 1 out]
                "Init. return code" <- w1769
                n707 = Equal?(x=w1767, y=w1769) -> (x = y?=w1766:bool)
              }
              frame #1 {
                n708 = Wait (ms)(milliseconds to wait=u32 2000) -> ()  [unwired: 1 out]
              }
              frame #2 {
                w1771 = u16 0  # ReadMode
                n709 = call "SetReadMode.vi"("mode"=w1771) -> ()  [unwired: 1 in, 2 out]
              }
              frame #3 {
                w1772 = u16 1  # AcquisitionMode
                n710 = call "SetAcquisitionMode.vi"("mode"=w1772) -> ()  [unwired: 1 in, 2 out]
              }
              frame #4 {
                w1773 = 0
                n711 = call "SetHSSpeed.vi"("index"=w1773, "type"=w1773) -> ()  [unwired: 2 in, 2 out]
              }
              frame #5 {
                n712 = call "GetNumberVSSpeeds.vi"() -> ("number"=w1776:i32)  [unwired: 3 in, 2 out]
                n713 = Subtract(x=w1776, y=1) -> (x-y=w1774:i32)
                n714 = call "SetVSSpeed.vi"("index"=w1774) -> ()  [unwired: 1 in, 2 out]
              }
              frame #6 {
                n715 = call "GetDetector.vi"() -> ("ypixels"=w1777:i32, "xpixels"=w1778:i32)  [unwired: 4 in, 2 out]
                "xpixels" <- w1778
                "ypixels" <- w1777
              }
            }
            n716 = flat-sequence {
              tunnel: w1710 -> [w1762]
              tunnel: [w1761] -> w1709
              frame #0 {
                n717 = case shown="False" w1762 {
                  selector: w1762 -> [w1764 w1765]
                  tunnel: [w1763 w1765] -> w1761
                  frame False {
                    n718 = Not(x=w1764) -> (.not. x?=w1763:bool)
                    n719 = call "Display Message to User5"() -> ()  [unwired: 10 in, 2 out]
                    n720 = Stop(stop? (T)=w1763) -> ()
                  }
                  frame True {
                  }
                }
              }
            }
            n721 = flat-sequence {
              tunnel: w1709 -> [w1718]
              tunnel: [w1716] -> w1706
              tunnel: w1705 -> [w1716]
              tunnel: [w1715] -> _
              frame #0 {
                w1719 = 36  # DRV_TEMP_STABILIZED
                w1720 = 20002  # DRV_SUCCESS
                # "set T ok?"
                # "timings ok?"
                n722 = stacked-sequence {
                  seq-local: [_ _ w1723 _ _ _] -> [_ _ _ _ _ _]
                  seq-local: [_ _ _ w1731 _ _] -> [_ _ _ _ w1735 w1736]
                  tunnel: w1720 -> [_ _ w1725 w1734 _ _]
                  tunnel: "Temperature\n(degrees C)" -> [_ _ _ w1732 _ _]
                  tunnel: w1719 -> [_ _ _ _ _ w1737]
                  tunnel: w1718 -> [_ _ w1724 _ _ _]
                  tunnel: [_ _ _ _ _ w1736] -> w1715
                  frame #0 {
                    n723 = call "SetTriggerMode.vi"("mode"=TriggerMode_mode_typedef."Internal") -> ()  [unwired: 1 in, 2 out]
                  }
                  frame #1 {
                    n724 = property on="Exposure time (s)" class="DigNum (strict)"() -> ("Value"=w1722:dbl)  [unwired: 2 in, 2 out]
                    n725 = call "SetExposureTime.vi"("time"=w1722) -> ()  [unwired: 1 in, 2 out]
                  }
                  frame #2 {
                    n726 = case shown="True" w1724 {
                      tunnel: w1725 -> [_ w1729]
                      tunnel: [FALSE w1730] -> w1723
                      frame False {
                      }
                      frame True {
                        n727 = call "GetAcquisitionTimings.vi"() -> ("exposure"=→"Calculated exposure time":sgl, "DLL error code"=w1728:u32)  [unwired: 11 in, 3 out]
                        "Check timings return code" <- w1728
                        n728 = Equal?(x=w1729, y=w1728) -> (x = y?=w1730:bool)
                      }
                    }
                  }
                  frame #3 {
                    n729 = call "SetTemperature.vi"("temperature"=w1732) -> ("DLL error code"=w1733:u32)  [unwired: 1 in, 1 out]
                    "Set temprature\nreturn code" <- w1733
                    n730 = Equal?(x=w1734, y=w1733) -> (x = y?=w1731:bool)
                  }
                  frame #4 {
                    n731 = case shown="True" w1735 {
                      frame False {
                      }
                      frame True {
                        n732 = call "CoolerON.vi"() -> ()  [unwired: 2 in, 2 out]
                      }
                    }
                  }
                  frame #5 {
                    n733 = case shown="True" w1736 {
                      tunnel: w1737 -> [_ w1738]
                      frame False {
                      }
                      frame True {
                        n734 = while {
                          tunnel: w1738 -> [w1742]
                          stop <- w1739 continue-if-true
                          n735 = Wait Until Next ms Multiple(millisecond multiple=u32 500) -> ()  [unwired: 1 out]
                          n736 = call "GetTemperature.vi"() -> ("status"=w1740:T18, "temperature"=→"Curent Temp":i32)  [unwired: 4 in, 2 out]
                          n737 = Not Equal?(x=w1742, y=w1740) -> (x != y?=w1739:bool)
                        }
                      }
                    }
                  }
                }
              }
            }
            n738 = for {
              N: 1023 -> [_]
              tunnel: [w1712] -> w1703 mode=indexing
              i -> [w1714]
              n739 = Add(x=1, y=w1714) -> (x+y=w1712:i32)
            }
            n740 = stacked-sequence {
              seq-local: [w1745 _ _] -> [_ w1750 _]
              tunnel: TRUE -> [w1744 _ _]
              tunnel: w1706 -> [_ _ w1759]
              tunnel: w1703 -> [_ _ w1757]
              frame #0 {
                n741 = case shown="True" w1744 {
                  tunnel: [FALSE w1749] -> w1745
                  frame False {
                  }
                  frame True {
                    w1747 = 20002  # DRV_SUCCESS
                    n742 = call "StartAcquisition.vi"() -> ("DLL error code"=w1748:u32)  [unwired: 2 in, 1 out]
                    "Start Aquisition return code" <- w1748
                    n743 = Equal?(x=w1747, y=w1748) -> (x = y?=w1749:bool)
                  }
                }
              }
              frame #1 {
                n744 = case shown="True" w1750 {
                  frame False {
                  }
                  frame True {
                    n745 = while {
                      stop <- w1753 continue-if-true
                      w1752 = u16 72  # DRV ACQUIRING
                      n746 = call "GetStatus.vi"() -> ("status"=w1751:T18)  [unwired: 3 in, 2 out]
                      n747 = Wait Until Next ms Multiple(millisecond multiple=u32 50) -> ()  [unwired: 1 out]
                      n748 = property on="Get status return code" class="DigNum (strict)"("Value"=w1751) -> ()  [unwired: 2 in, 2 out]
                      n749 = Equal?(x=w1751, y=w1752) -> (x = y?=w1753:bool)
                    }
                  }
                }
              }
              frame #2 {
                n750 = call "GetAcquiredData.vi"("size"=w1759) -> ("DLL error code"=→"get aquired data return code":u32, "array"=w1756:i32[])  [unwired: 2 in, 1 out]
                n751 = Bundle(w1757, "array"=w1756) -> (→"?":cluster{i32[], "array":i32[]})  [unwired: 1 in]
                "T reached?" <- TRUE ("T reached?")
              }
            }
          }
          frame True {
            n752 = property on="T reached?" class="Bool (strict)"("Value"=FALSE ("T reached?")) -> ()  [unwired: 2 in, 2 out]
            n753 = stacked-sequence {
              frame #0 {
                n754 = call "CoolerOFF.vi"() -> ("DLL error code"=→"Cooler Off return code":u32)  [unwired: 2 in, 1 out]
              }
              frame #1 {
                n755 = while {
                  stop <- w1784 continue-if-true
                  n756 = call "GetTemperature.vi"() -> ("temperature"=w1782:i32)  [unwired: 4 in, 3 out]
                  n757 = property on="Curent Temp" class="DigNum (strict)"("Value"=w1782) -> ()  [unwired: 2 in, 2 out]
                  n758 = Less?(x=w1782, y=i16 0) -> (x < y?=w1784:bool)
                  n759 = Wait Until Next ms Multiple(millisecond multiple=u32 500) -> ()  [unwired: 1 out]
                }
              }
              frame #2 {
                n760 = call "ShutDown.vi"() -> ()  [unwired: 2 in, 2 out]
                "Shut down sequence run?" <- TRUE ("Shut down complete?")
              }
            }
          }
        }
      }
    }
    n761 = property on="Use autolab?" class="Bool (strict)"() -> ("Value"=w4:bool)  [unwired: 2 in, 2 out]
    n762 = Equal To 0?(x=w22) -> (x = 0?=w30:bool)
    n763 = case shown="True" w4 {
      tunnel: w31 -> [w47 w83]
      tunnel: w30 -> [w46 _]
      tunnel: [w45 w83] -> w24
      tunnel: [w42 FALSE] -> w20
      frame False {
        n764 = case shown="False" w46 {
          tunnel: w47 -> [w56 w82]
          tunnel: [w55 w80] -> w45
          tunnel: [w50 w74] -> w39
          tunnel: [w51 w75] -> w43
          tunnel: [w53 w81] -> w41
          tunnel: [w49 w73] -> w40
          tunnel: [w52 w76] -> w44
          frame False {
            n765 = call "IV getcellstatus.vi"() -> ("devcellstatus out"=w66:i32)  [unwired: 9 in, 2 out]
            n766 = call "Bitget 8-bits test.vi"("x"=w66) -> ("c"=w62:dbl, "e"=w64:dbl, "f"=w63:dbl, "h"=w65:dbl)  [unwired: 19 in, 4 out]
            n767 = Greater?(x=w62, y=0.0) -> (0:w68:bool)
            n768 = Greater?(x=w64, y=0.0) -> (0:w69:bool)
            n769 = Greater?(x=w63, y=0.0) -> (0:w70:bool)
            n770 = Greater?(x=w65, y=0.0) -> (0:w48:bool)
            n771 = And(x=w66, y=256) -> (x .and. y?=w67:i32)
            n772 = Equal?(x=w67, y=256) -> (x = y?=w71:bool)
            n773 = Bundle By Name(cluster=w56, "I overload"=w68, "Aninput1 overload"=w69, "E overload"=w70, "Cell of button pressed"=w48, "Cell on"=w71) -> (w55:T11)
            n774 = Unbundle By Name(w55) -> ("I overload"=w53:bool, "Aninput1 overload"=w52:bool, "E overload"=w51:bool, "Cell of button pressed"=w50:bool, "Cell on"=w49:bool)
          }
          frame True {
            w72 = FALSE
            # "After closing the driver reset the indicators"
            n775 = property class="XYGraph (strict)"("Value"=cluster{dbl[], dbl[]} {[], []} ("XY Graph")) -> ()  [unwired: 2 in, 2 out]
            n776 = property on="Potentiostat Status" class="Str"("Value"="" ("Device Status indicator")) -> ()  [unwired: 2 in, 2 out]
            n777 = property on="Device serial number" class="Str"("Value"="" ("Device serial number")) -> ()  [unwired: 2 in, 2 out]
            n778 = Bundle By Name(cluster=w82, "I overload"=w72, "Aninput1 overload"=w72, "E overload"=w72, "Cell of button pressed"=w72, "Cell on"=w72) -> (w80:T11)
            n779 = Unbundle By Name(w80) -> ("I overload"=w81:bool, "Aninput1 overload"=w76:bool, "E overload"=w75:bool, "Cell of button pressed"=w74:bool, "Cell on"=w73:bool)
          }
        }
        "I_overload" <- w41
        "Aninput1_overload" <- w44
        "E_overload" <- w43
        "cell-off button pressed" <- w39
        "cell on" <- w40
        n780 = Or(x=w41, y=w43) -> (x .or. y?=w42:bool)
      }
      frame True {
      }
    }
    n781 = Unbundle By Name(w31) -> ("Current"=→"current":dbl, "Serial No"=→"Device serial number":string, "Status"=→"Potentiostat Status":string)
    n782 = Or(x=w25, y=w36) -> (x .or. y?=w35:bool)
    n783 = case shown="False" w20 {
      tunnel: w7 -> [w85 w86]
      tunnel: [w85 w86] -> w21
      frame False {
      }
      frame True {
        n784 = disable-structure shown="Disabled" {
          disable-tunnel: [State."Exit" ("f") _] -> _
          frame Disabled {
            n785 = call "Display Message to User"() -> ()  [unwired: 10 in, 2 out]
          }
          frame Enabled {
          }
        }
      }
    }
  }
